vi "Time.vi"(8 "error in (no error)":errorcluster, 10 "Control In":T2={"I-O.lvclass"=refnum, "Gantry"=refnum, "Dispenser"="COM1"}, 11 "Sensor Dispense in":refnum<class "Sensor Dispense.lvclass">) -> (0 "error out":errorcluster, 1 "Timing Data":i32[](array[numeric]), 2 "Control Out":T2={"I-O.lvclass"=refnum, "Gantry"=refnum, "Dispenser"="COM1"}, 3 "Sensor Dispense out":refnum<class "Sensor Dispense.lvclass">)   [LabVIEW 2021, in "Sensor Dispense.lvclass"]
uses:
  Projects/Sensor Dispense.lvclass
  C:/Users/hep/Documents/UCSB-CMU-GantryCode/UCSB-Gantry-HEP-main (3)/UCSB-Gantry-HEP-main/Classes/Routine/Dispense/Dispense.lvclass
  Controller/Controllers.ctl
  Controller/I-O/I-O.lvclass
  C:/Program Files (x86)/Aerotech/A3200/LabVIEW/2010/Bin/Aerotech.A3200.dll
  Program Files (x86)/Aerotech/A3200/LabVIEW/2010/Bin/Aerotech.A3200.dll
  TypeOfHexaboard.ctl
  Projects/Sensor Dispense.lvclass/Sensor Dispense.ctl
  Controller/Motion/Motion.lvclass
  Controller/Motion/A3200/A3200.lvclass
  Controller/Controller.lvclass
  Routine.lvclass
panel:
  in  "Type of Hexaboard":T1
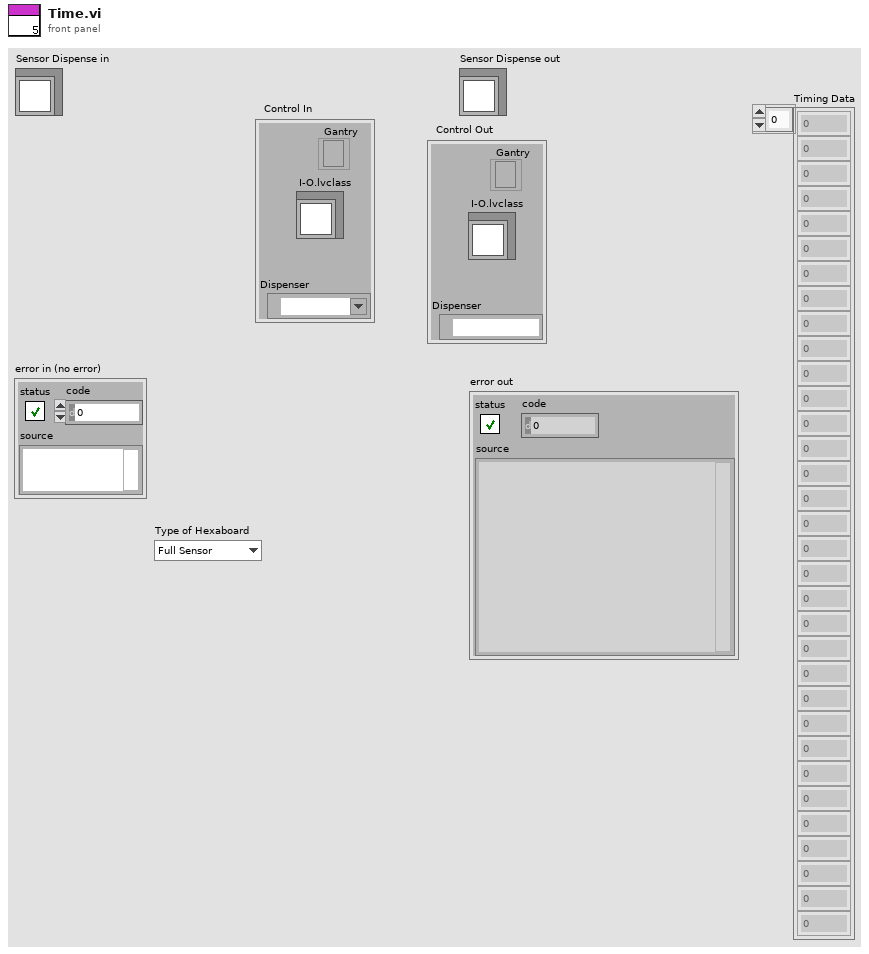
[diagram p1: front panel]
types:
  T1 = typedef "Routine.lvclass/TypeOfHexaboard.ctl" = enum16{"Full Sensor", "Full PCB", "Right Partial PCB", "Right Partial Sensor", "Al Dummy Right Partial Sensor"}
  T2 = typedef "Controller.lvclass/Controllers.ctl" = cluster{"I-O.lvclass":refnum<class "I-O.lvclass">, "Gantry":refnum<k24>, "Dispenser":refnum<visa-resource-name>}
  T3 = cluster{"Endpoints":dbl[][], "Center":dbl[], "CW/CCW":dbl, "Dispense Type":enum16{"N-gon", "Square", "Arc", "Dot", "Line", "Circle"}}[]
  T4 = cluster{"Endpoints":dbl[][], "Center":dbl[], "CW/CCW":dbl, "Dispense Type":enum16{"N-gon", "Square", "Arc", "Dot", "Line", "Circle"}}
  T5 = enum16{"N-gon", "Square", "Arc", "Dot", "Line", "Circle"}
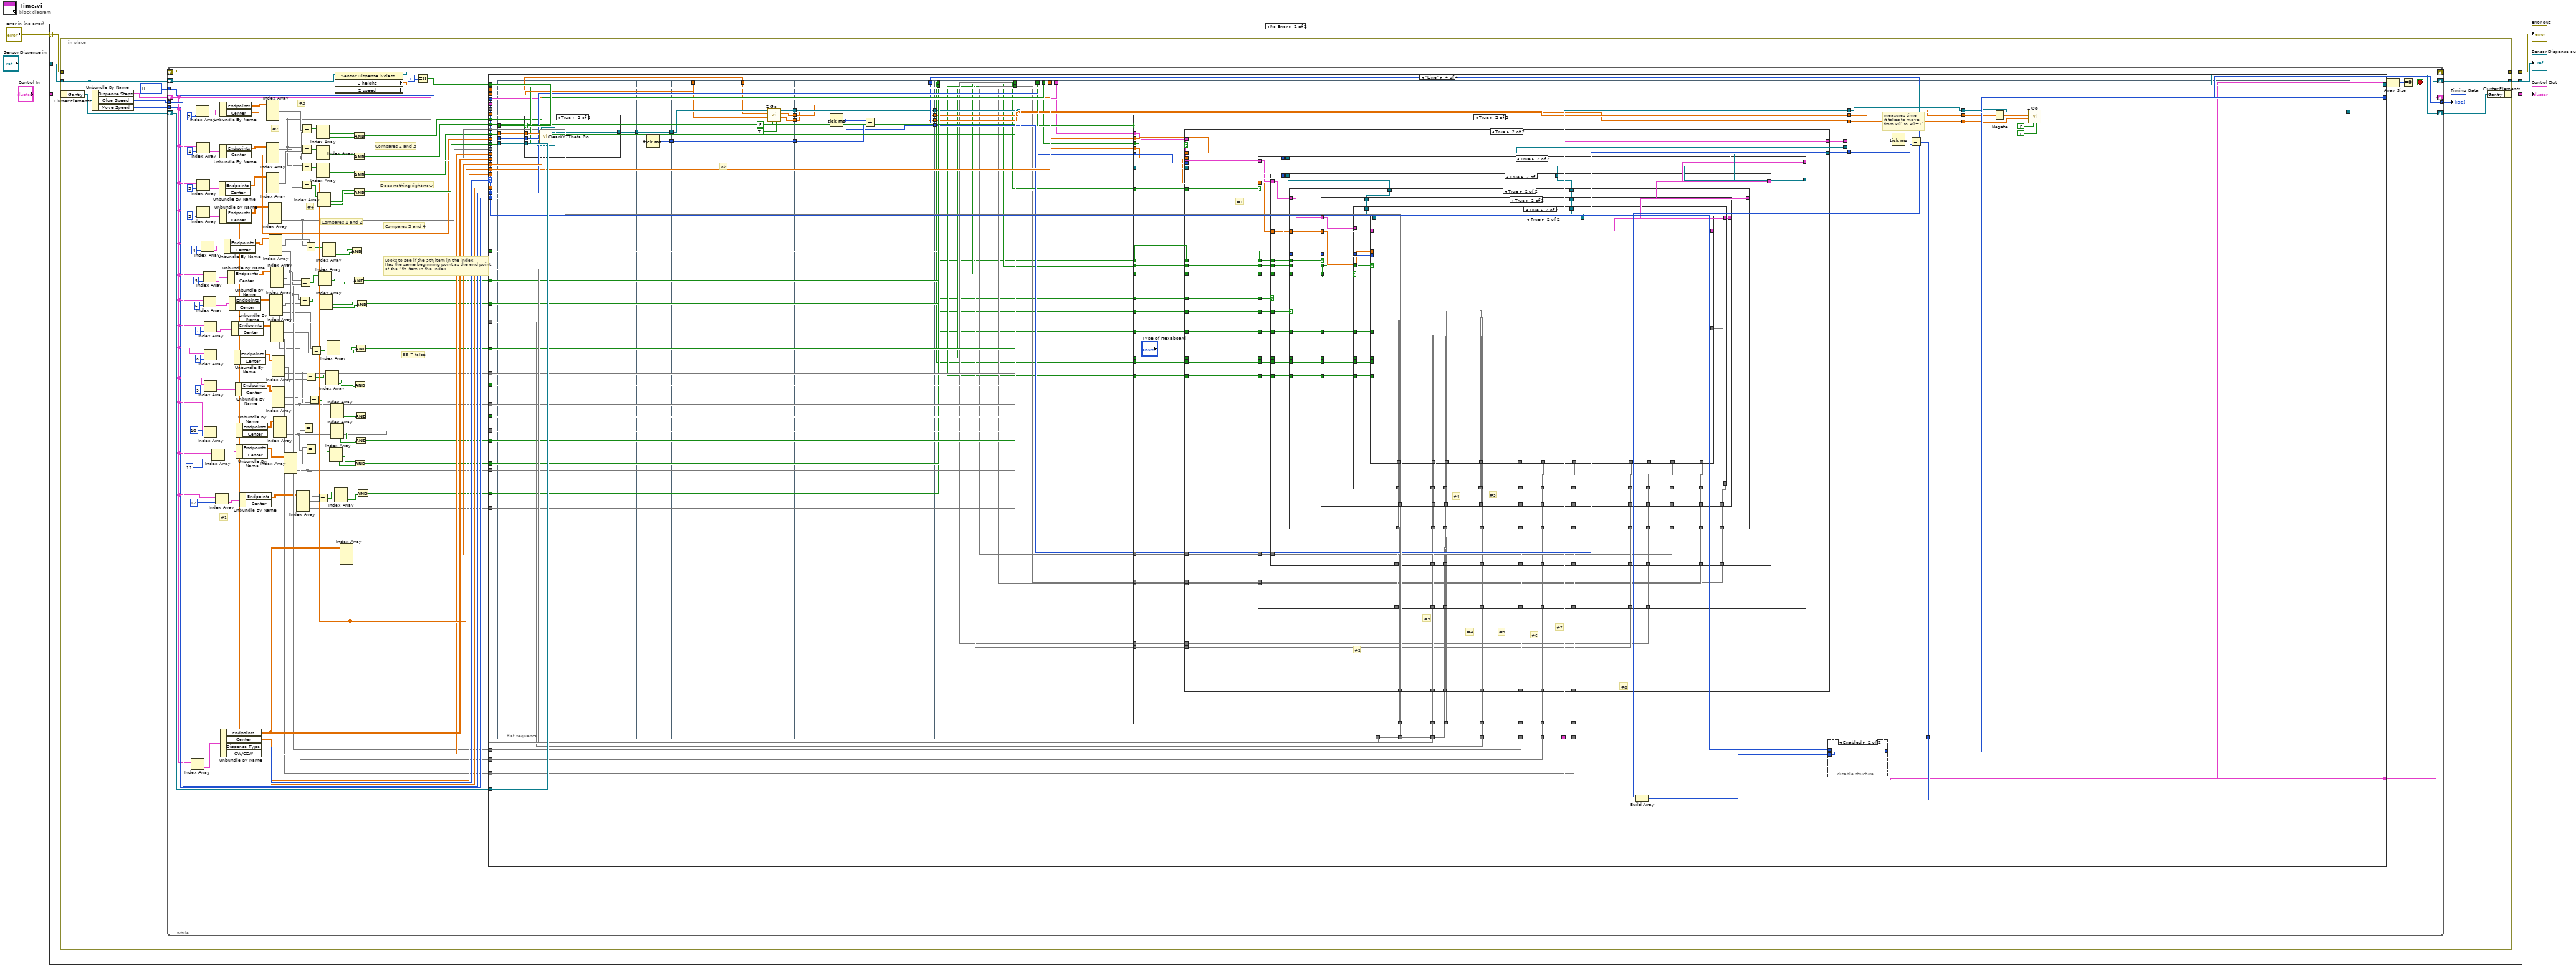
[diagram p0: block diagram]
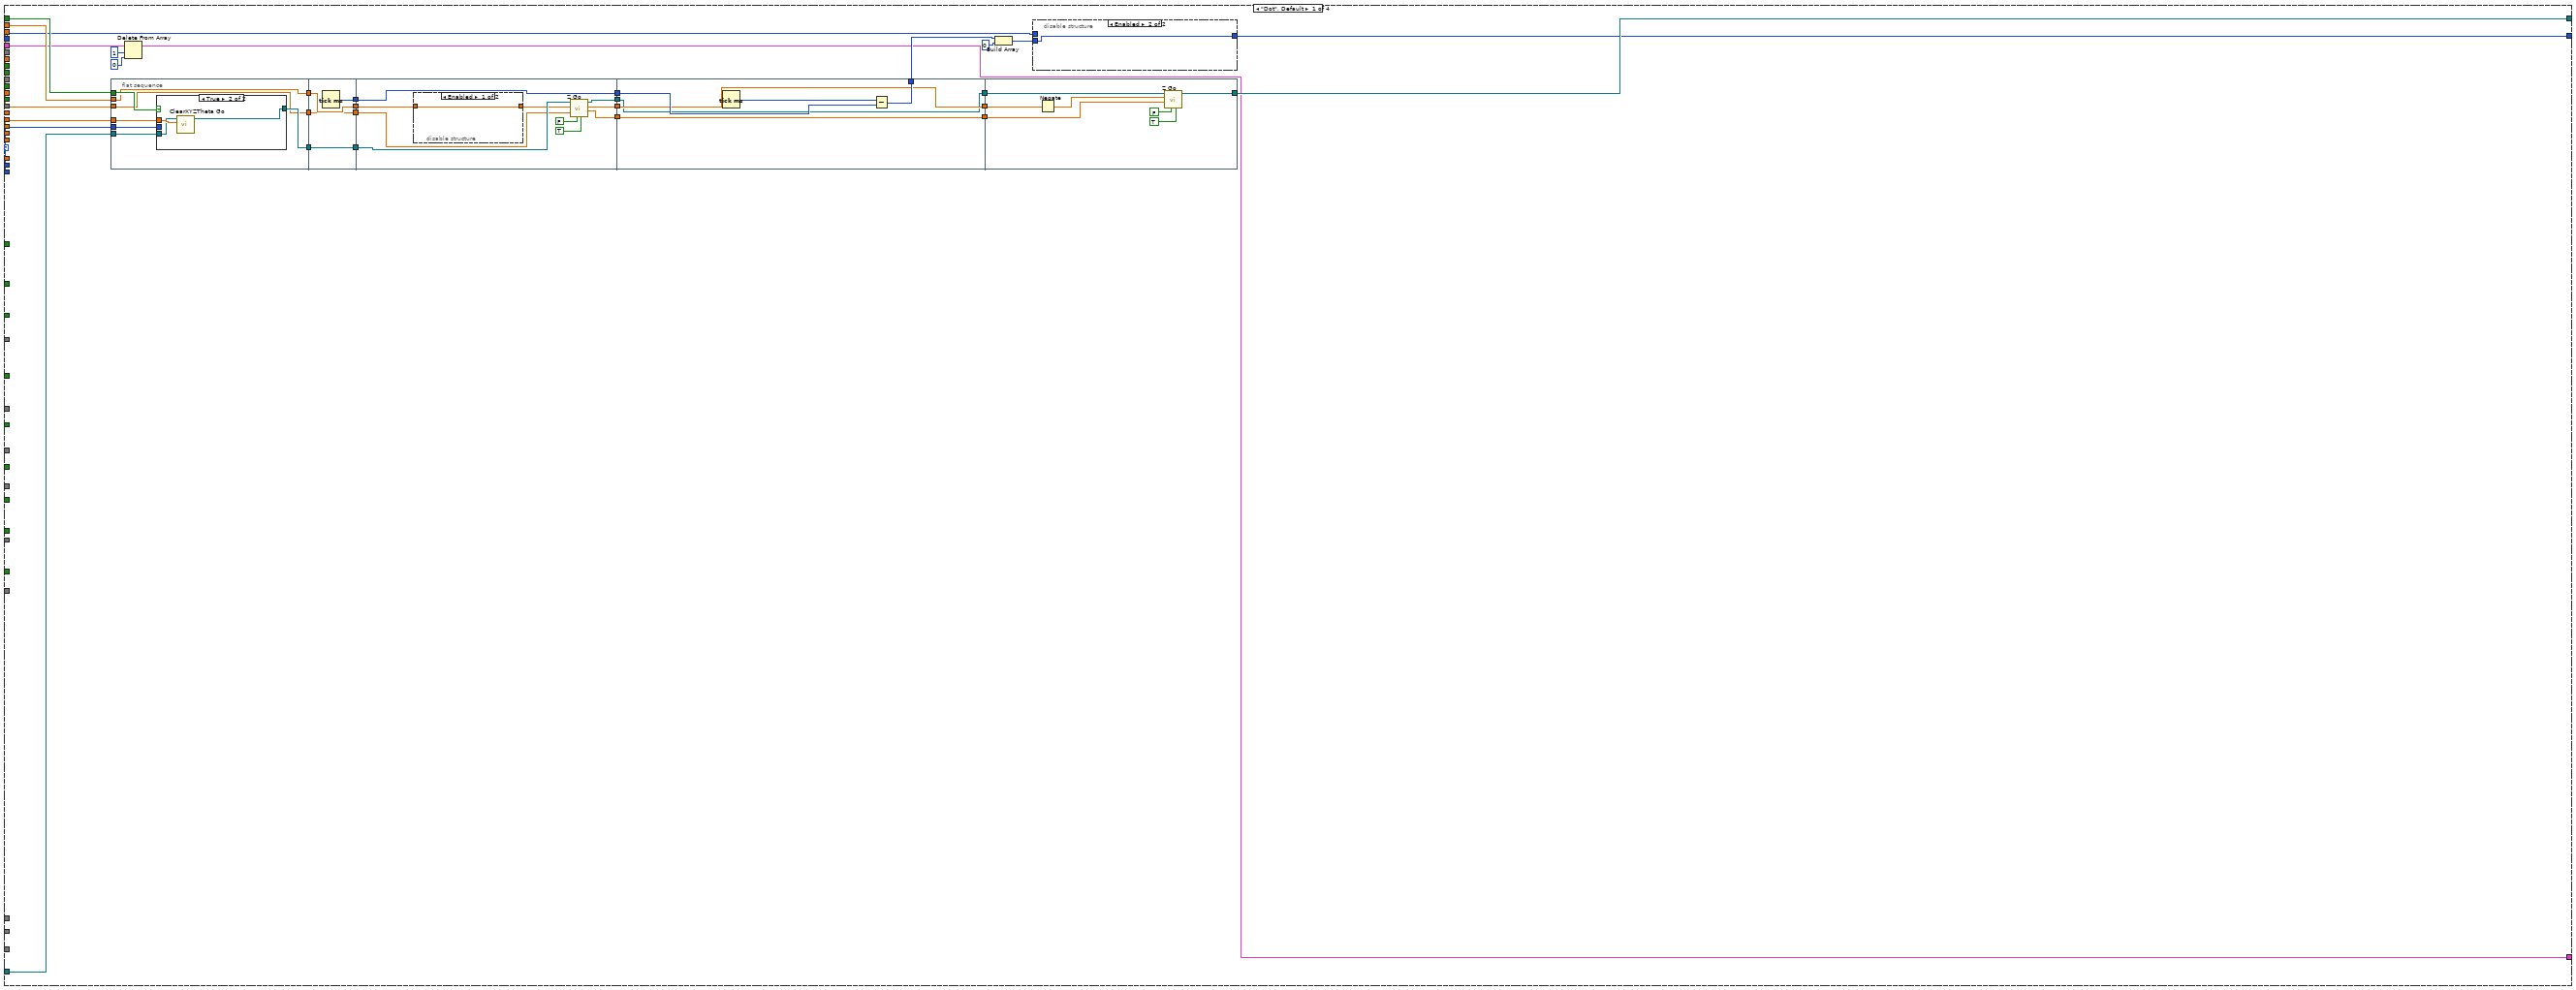
[diagram p2: hidden frame]
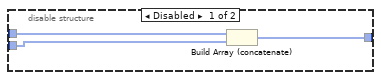
[diagram p3: hidden frame]
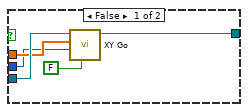
[diagram p4: hidden frame]
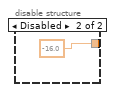
[diagram p5: hidden frame]
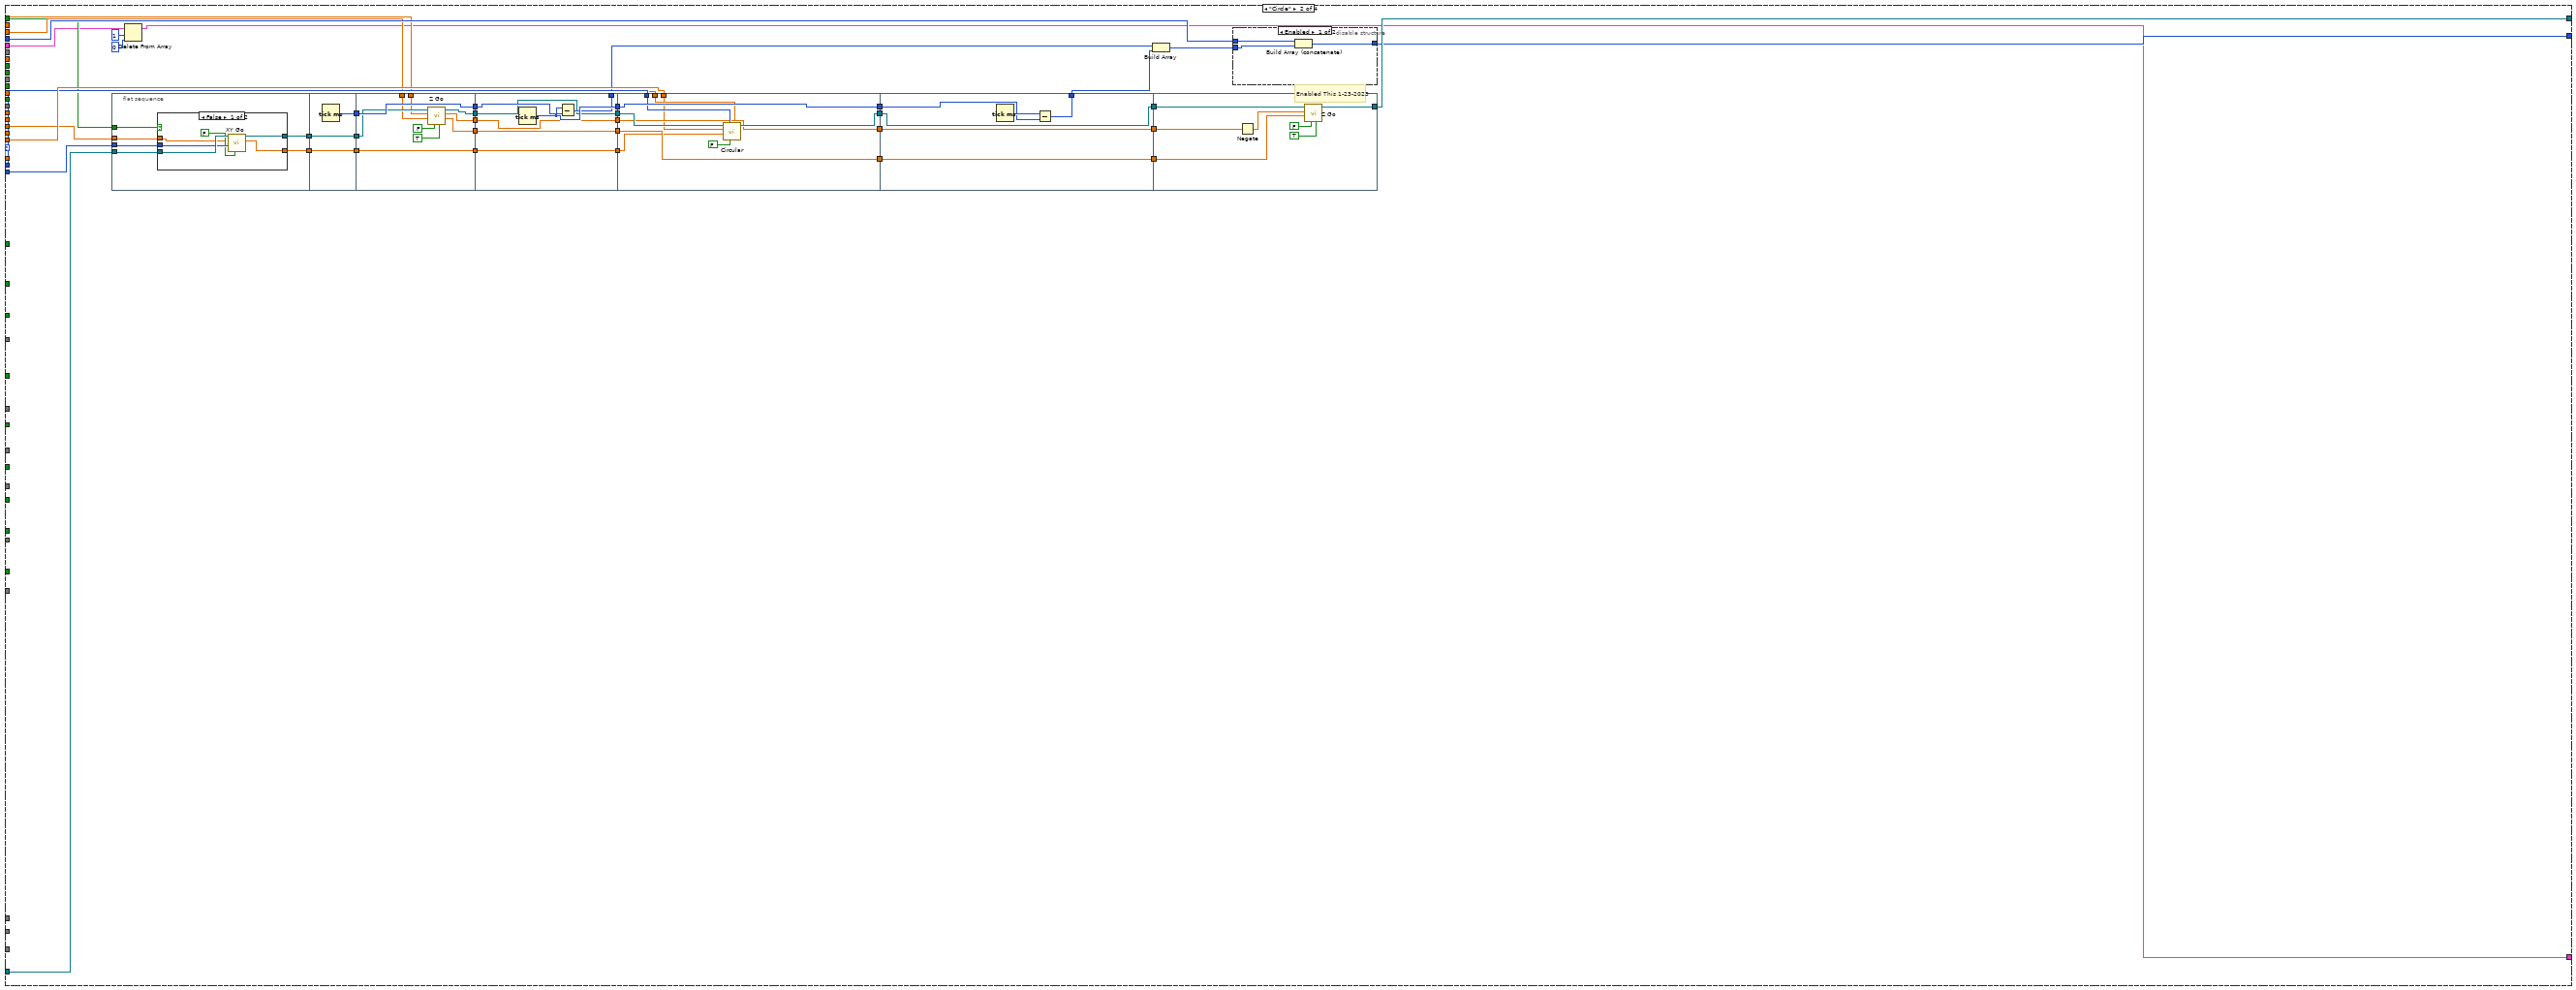
[diagram p6: hidden frame]
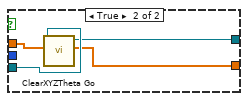
[diagram p8: hidden frame]
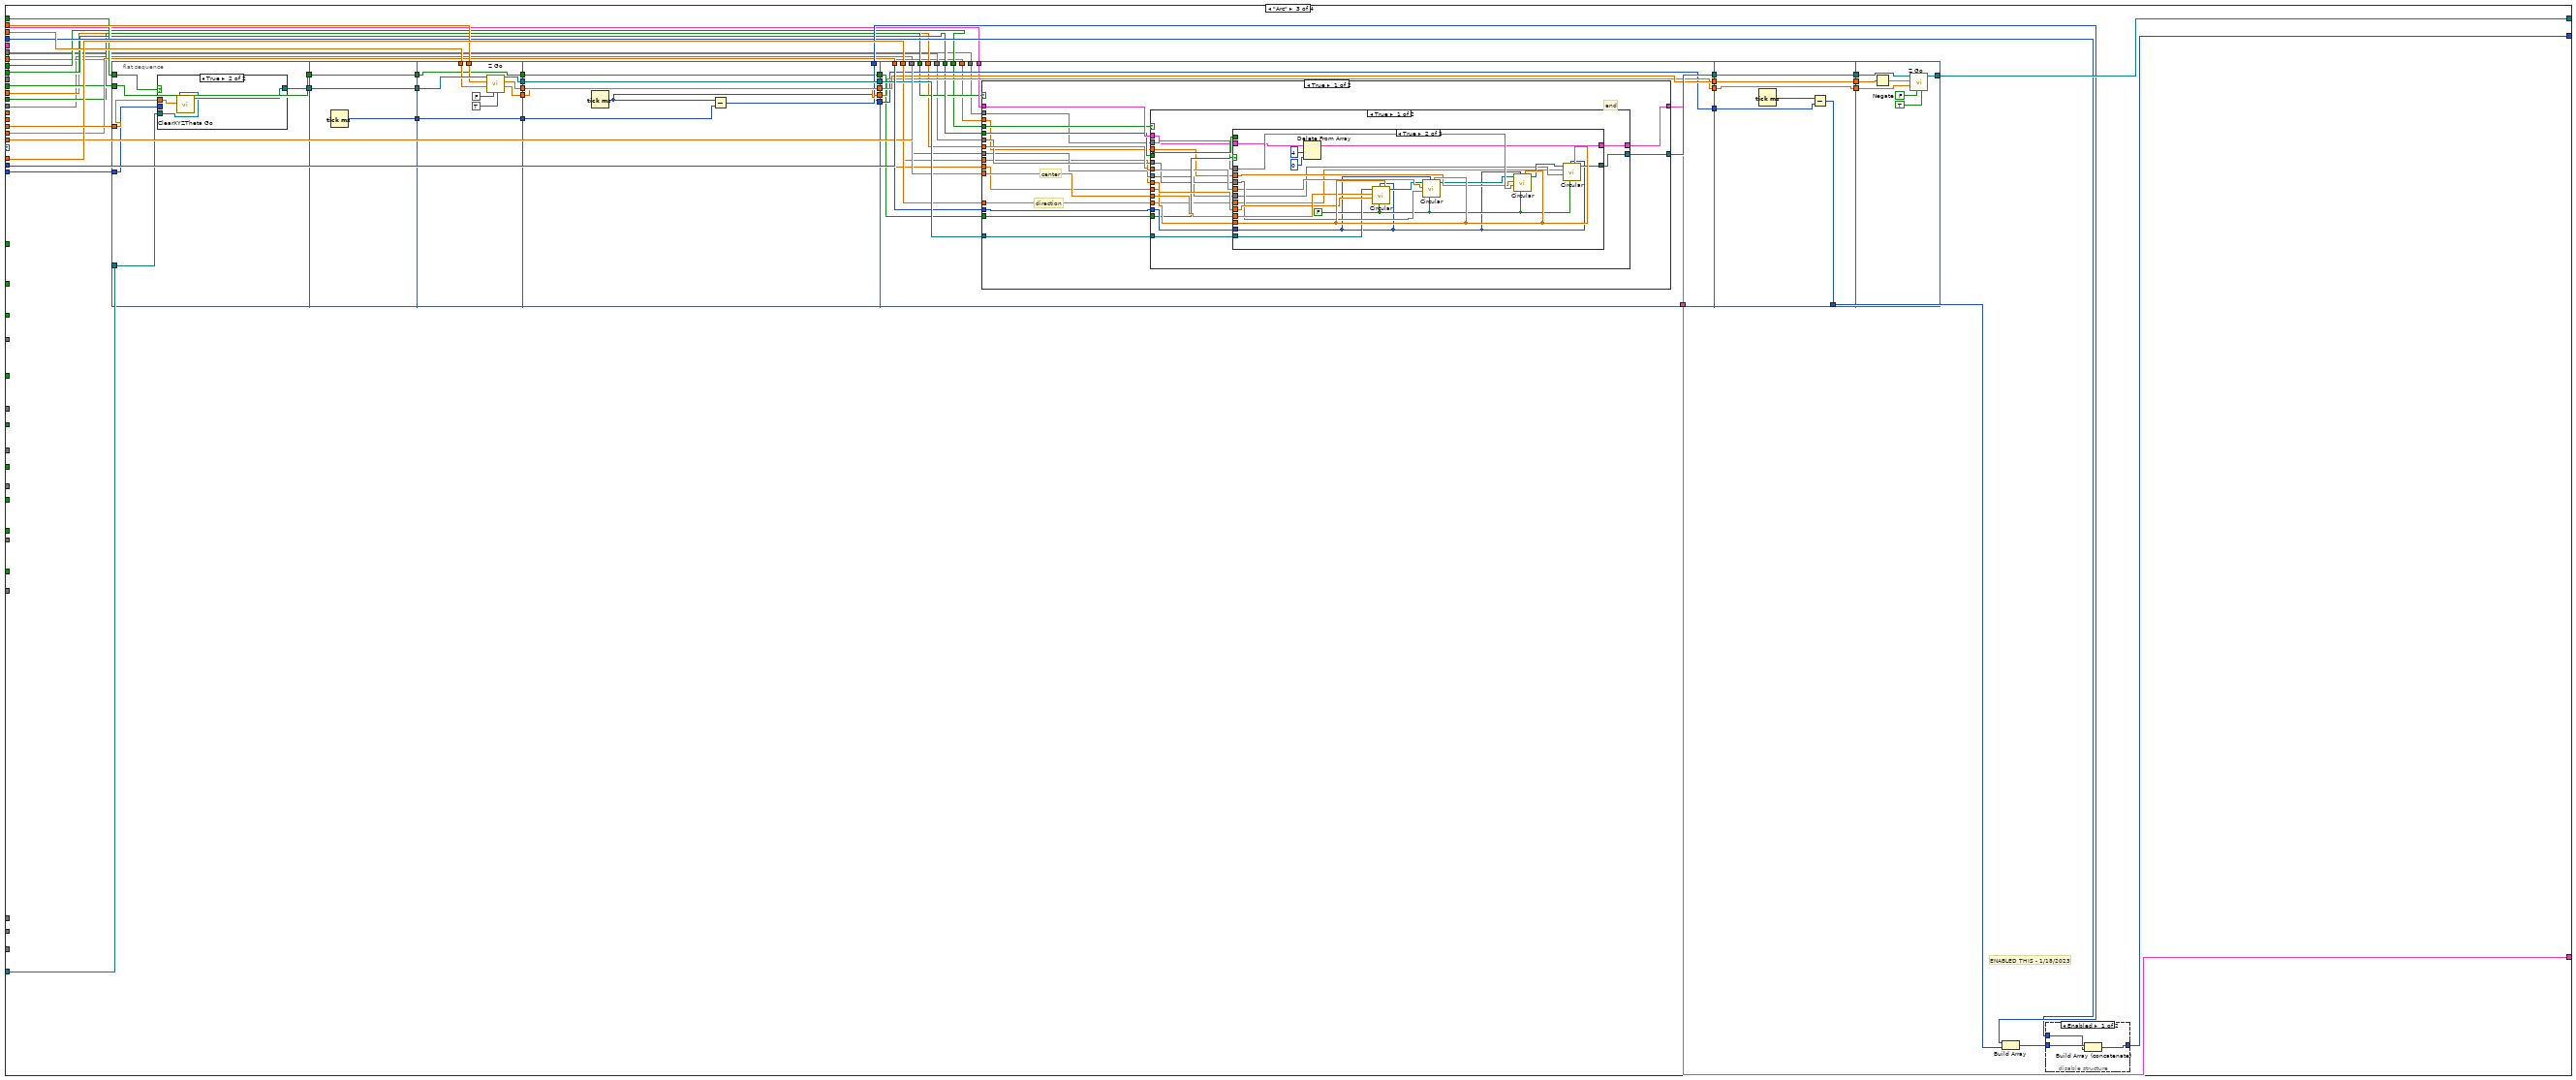
[diagram p9: hidden frame]
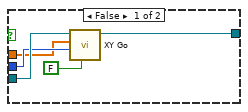
[diagram p11: hidden frame]
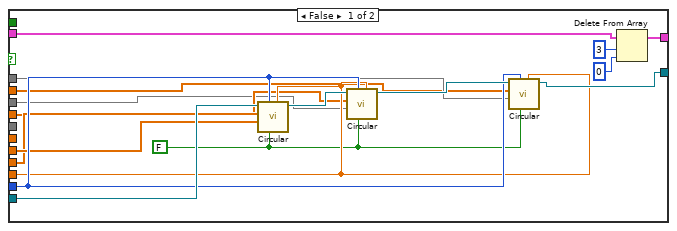
[diagram p12: hidden frame]
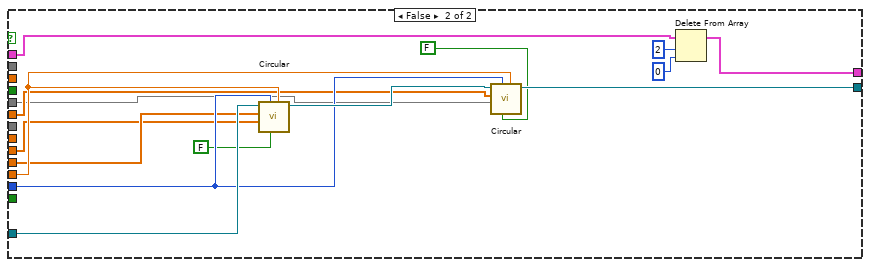
[diagram p13: hidden frame]
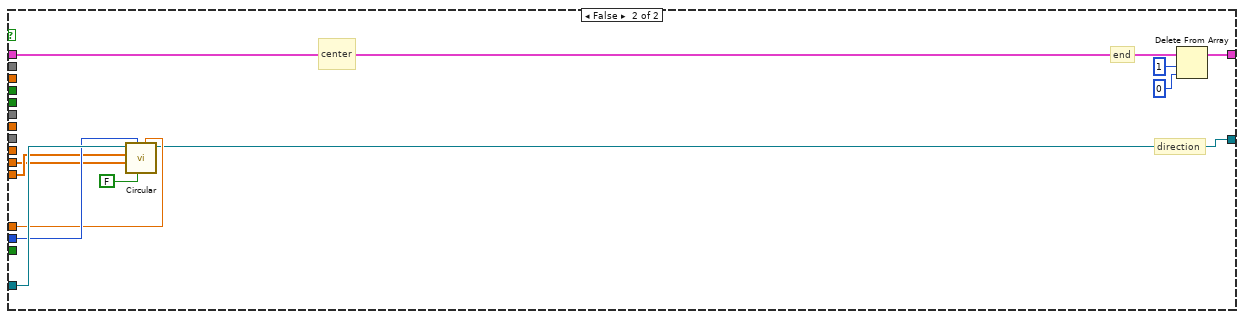
[diagram p14: hidden frame]
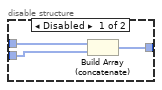
[diagram p15: hidden frame]
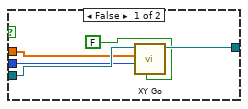
[diagram p16: hidden frame]
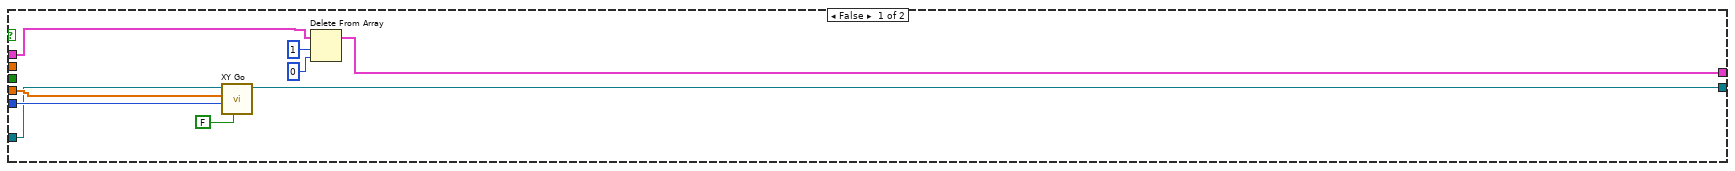
[diagram p17: hidden frame]
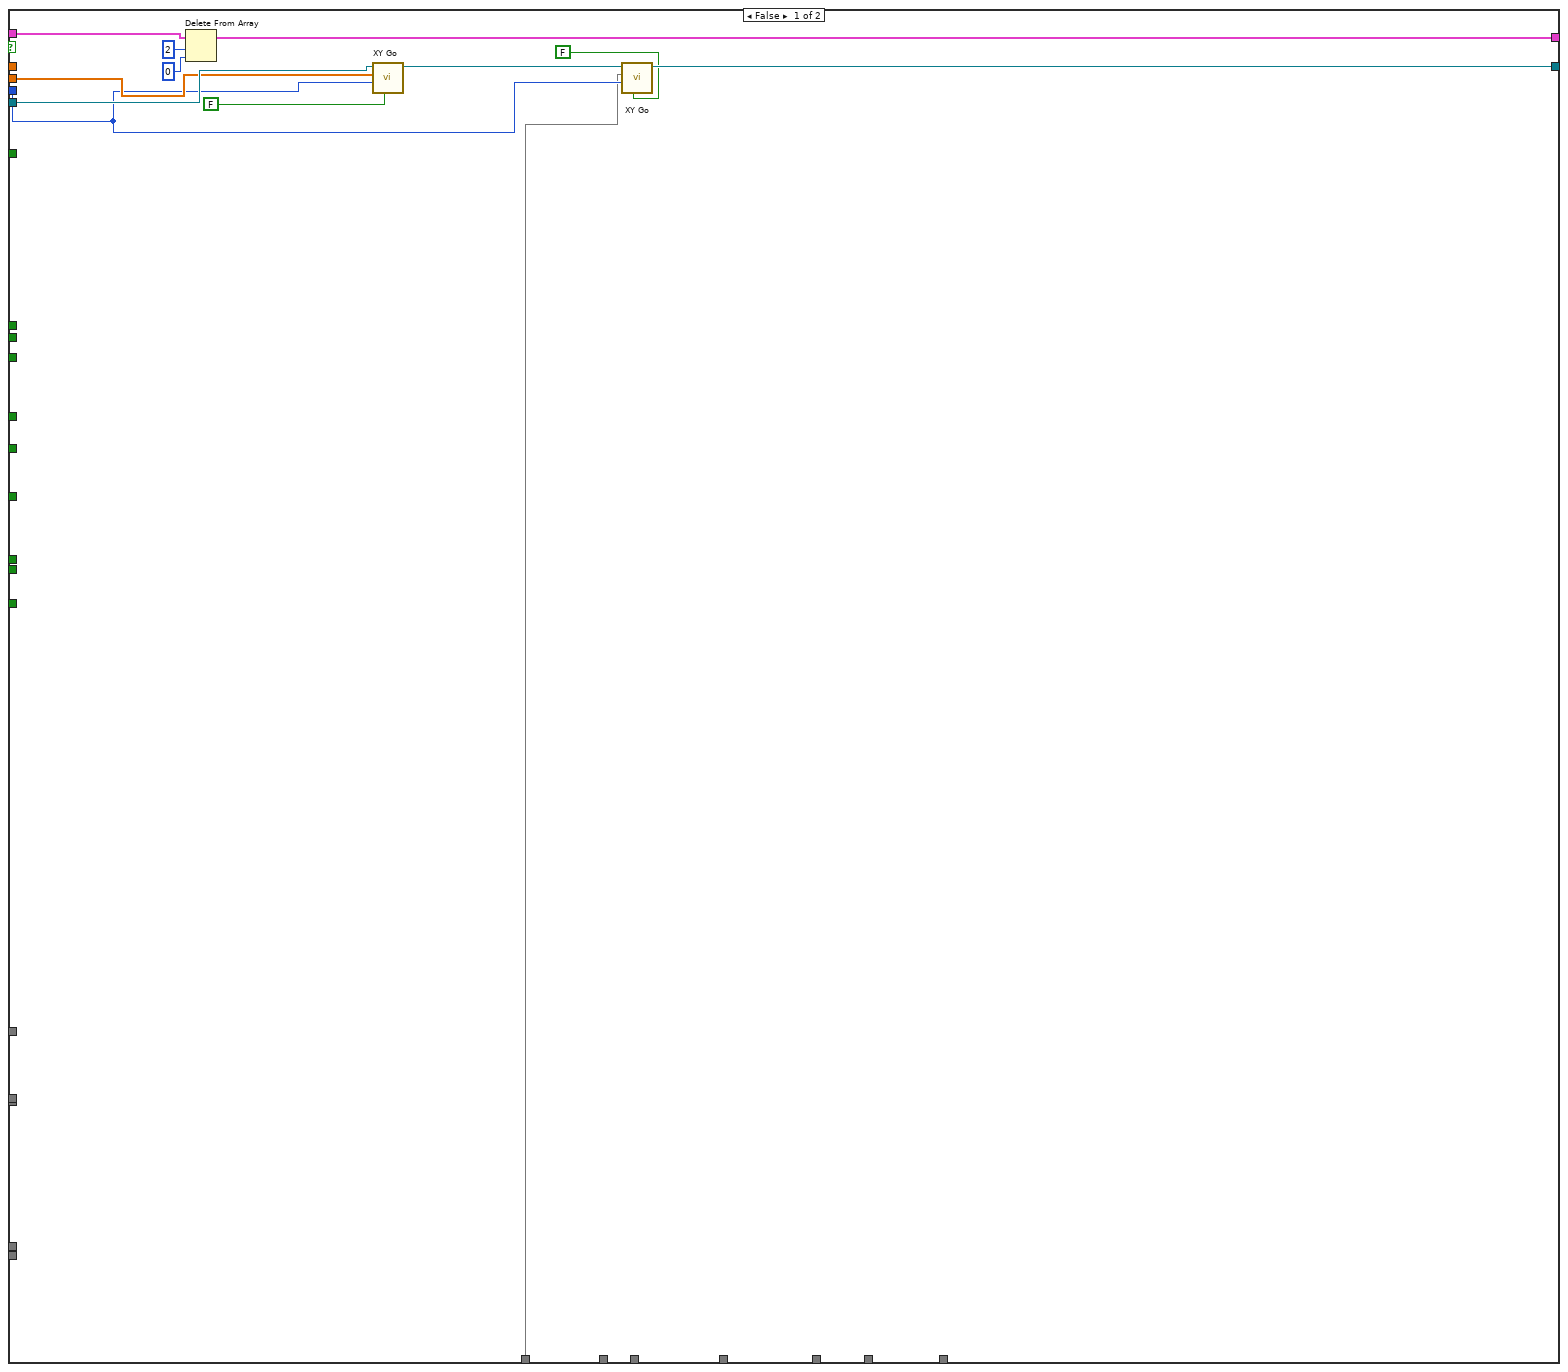
[diagram p18: hidden frame]
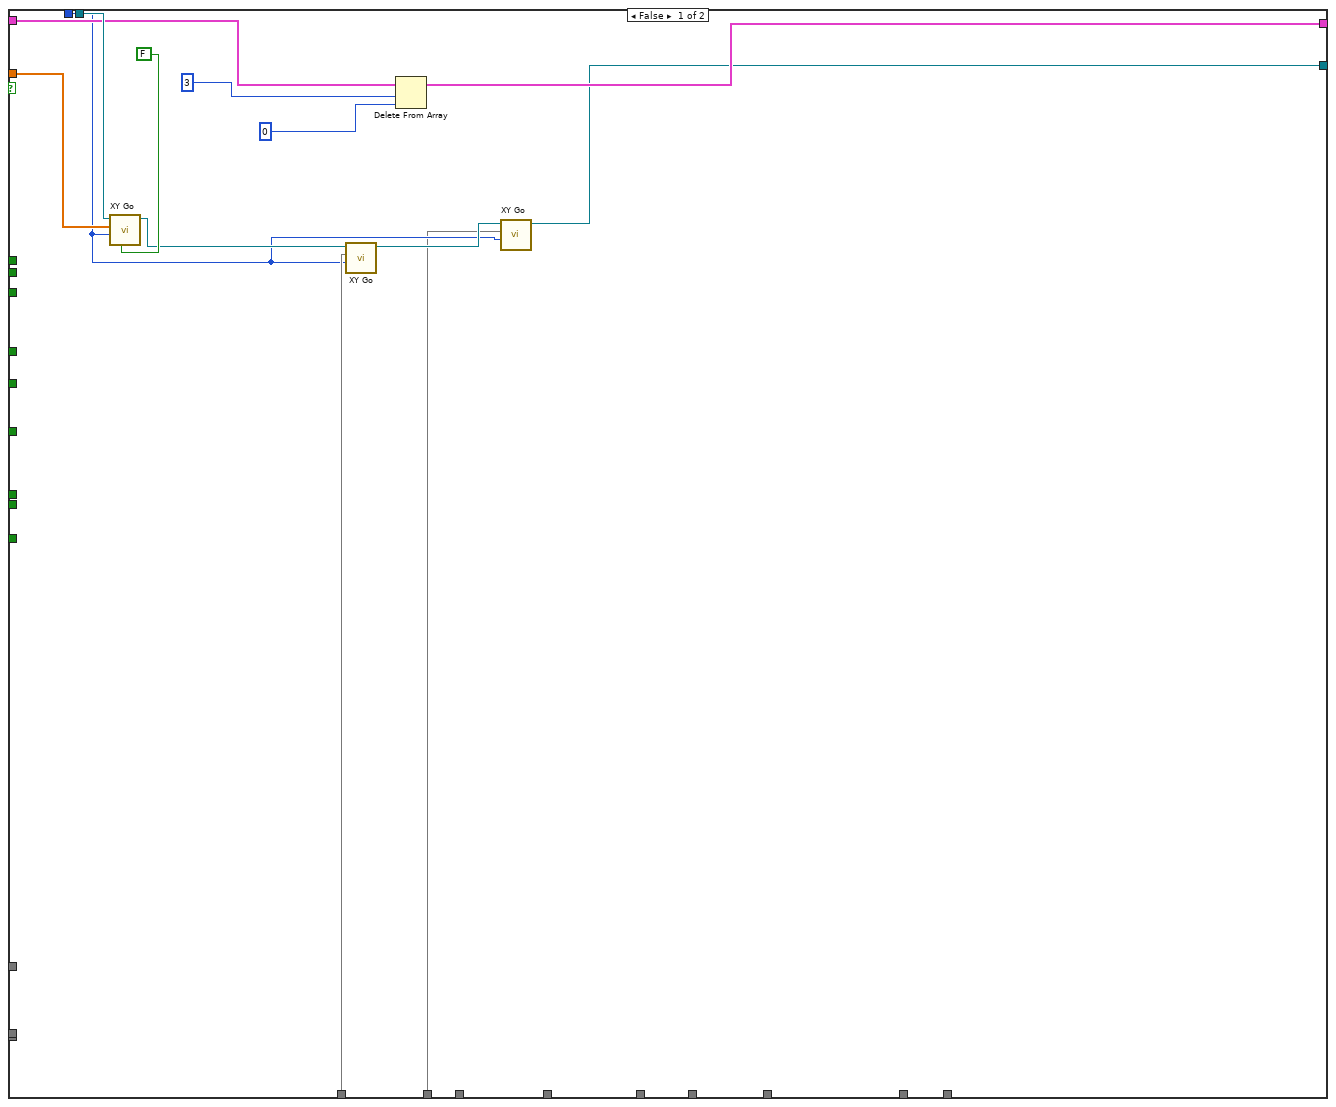
[diagram p19: hidden frame]
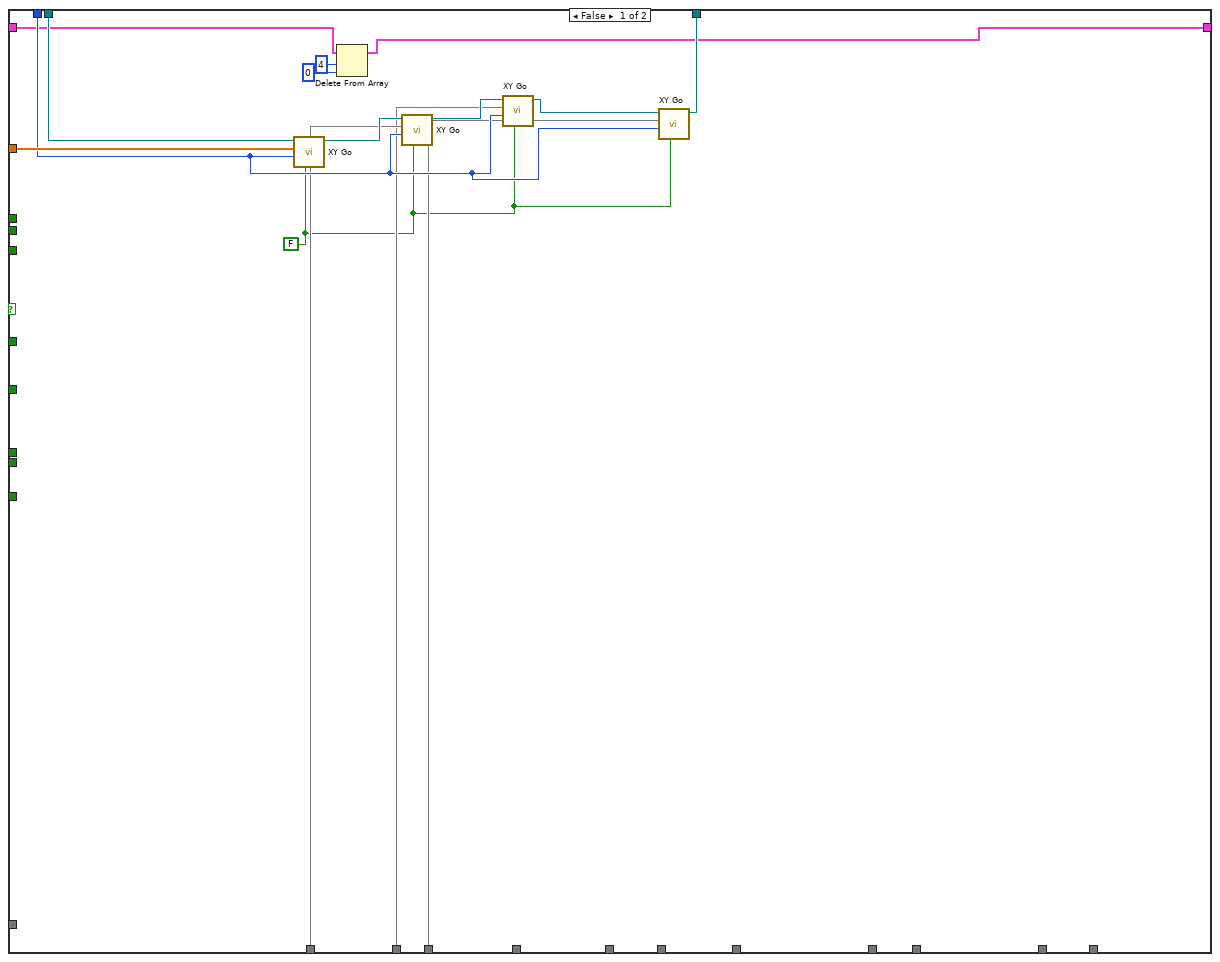
[diagram p20: hidden frame]
diagram:
  n1 = case shown="No Error" "error in (no error)" {
    selector: "error in (no error)" -> [w7 w1242]
    tunnel: "Sensor Dispense in" -> [w12 w1240]
    tunnel: [w11 w1240] -> w5
    tunnel: "Control In" -> [w10 w1241]
    tunnel: [w9 w1241] -> w3
    tunnel: [w8 w1242] -> w2
    frame No Error {
      n2 = in-place {
        in-place-border: w12 -> [w21]
        in-place-border: [w20] -> w11
        in-place-border: [w16] -> w8
        in-place-border: w7 -> [w15]
        n3 = in-place-cluster #1(w10) -> ("Gantry"=w22:refnum<k24>)
        n4 = Unbundle By Name "Unbundle By Name"(w21) -> ("Dispense Steps"=w17:T3, "Glue Speed"=w13:i32, "Move Speed"=w14:i32)
        n5 = while {
          tunnel: w14 -> [w166]
          shift-right: [w155] -> w19
          shift-left: w22 -> [w164]
          tunnel: w13 -> [w152]
          shift-right: [w162] -> w20
          shift-left: w21 -> [w163]
          shift-right: [w113] -> w16
          shift-left: w15 -> [w113]
          tunnel: i32[] [] -> [w165]
          tunnel: [w157] -> w18 mode=concatenating
          shift-right: [w115] -> _
          shift-left: w17 -> [w40]
          i -> [w161]
          stop <- w112 stop-if-true
          # "85 = false"
          # "Looks to see if the 5th item in the index\nHas the same beginning point as the end point\nof the 4th item in the index"
          # "Does nothing right now"
          # "Compares 2 and 3"
          # "Compares 3 and 4"
          # "Compares 1 and 2"
          # "#3"
          # "#2"
          # "#1"
          # "#4"
          n6 = Index Array(array=w40) -> (element=w148:T4)  [unwired: 1 in]
          n7 = Index Array "Index Array"(array=w40, index=2) -> (element=w146:T4)
          n8 = Index Array(array=w40, index=1) -> (element=w145:T4)
          n9 = Index Array(array=w40, index=3) -> (element=w147:T4)
          n10 = Index Array(array=w40, index=3) -> (element=w150:T4)
          n11 = Index Array "Index Array"(array=w40, index=4) -> (element=w105:T4)
          n12 = Index Array "Index Array"(array=w40, index=5) -> (element=w93:T4)
          n13 = Index Array "Index Array"(array=w40, index=6) -> (element=w94:T4)
          n14 = Index Array "Index Array"(array=w40, index=7) -> (element=w95:T4)
          n15 = Index Array "Index Array"(array=w40, index=8) -> (element=w70:T4)
          n16 = Index Array "Index Array"(array=w40, index=9) -> (element=w69:T4)
          n17 = Index Array "Index Array"(array=w40, index=10) -> (element=w68:T4)
          n18 = Index Array "Index Array"(array=w40, index=11) -> (element=w67:T4)
          n19 = Index Array "Index Array"(array=w40, index=12) -> (element=w66:T4)
          n20 = Unbundle By Name(w147) -> ("Endpoints"=w139:dbl[][])  [unwired: 1 out]
          n21 = Unbundle By Name(w146) -> ("Endpoints"=w140:dbl[][], "Center"=w117:dbl[])
          n22 = Unbundle By Name(w145) -> ("Endpoints"=w138:dbl[][], "Center"=w109:dbl[])
          n23 = Unbundle By Name(w150) -> ("Endpoints"=w141:dbl[][], "Center"=w116:dbl[])
          n24 = Unbundle By Name(w148) -> ("Endpoints"=w154:dbl[][], "Center"=w153:dbl[], "Dispense Type"=w156:T5, "CW/CCW"=w151:dbl)
          n25 = Unbundle By Name(w105) -> ("Endpoints"=w101:dbl[][])  [unwired: 1 out]
          n26 = Unbundle By Name(w93) -> ("Endpoints"=w92:dbl[][])  [unwired: 1 out]
          n27 = Unbundle By Name(w94) -> ("Endpoints"=w91:dbl[][])  [unwired: 1 out]
          n28 = Unbundle By Name(w95) -> ("Endpoints"=w90:dbl[][])  [unwired: 1 out]
          n29 = Unbundle By Name(w70) -> ("Endpoints"=w65:dbl[][])  [unwired: 1 out]
          n30 = Unbundle By Name(w69) -> ("Endpoints"=w60:dbl[][])  [unwired: 1 out]
          n31 = Unbundle By Name(w68) -> ("Endpoints"=w54:dbl[][])  [unwired: 1 out]
          n32 = Unbundle By Name(w67) -> ("Endpoints"=w48:dbl[][])  [unwired: 1 out]
          n33 = Unbundle By Name(w66) -> ("Endpoints"=w42:dbl[][])  [unwired: 1 out]
          n34 = Index Array(array=w140) -> (element #1=w130:dbl[], element #2=w118:dbl[])  [unwired: 4 in]
          n35 = Index Array(array=w138) -> (element #1=w121:dbl[], element #2=w111:dbl[])  [unwired: 4 in]
          n36 = Index Array(array=w139) -> (element #1=w134:dbl[])  [unwired: 4 in, 1 out]
          n37 = Index Array(array=w141) -> (element #1=w123:dbl[], element #2=w99:dbl[])  [unwired: 4 in]
          n38 = Index Array(array=w101) -> (element #1=w100:dbl[], element #2=w89:dbl[])  [unwired: 4 in]
          n39 = Index Array(array=w91) -> (element #1=w83:dbl[], element #2=w38:dbl[])  [unwired: 4 in]
          n40 = Index Array(array=w92) -> (element #1=w88:dbl[], element #2=w84:dbl[])  [unwired: 4 in]
          n41 = Index Array(array=w90) -> (element #1=w79:dbl[], element #2=w39:dbl[])  [unwired: 4 in]
          n42 = Index Array(array=w65) -> (element #1=w64:dbl[], element #2=w58:dbl[])  [unwired: 4 in]
          n43 = Index Array(array=w60) -> (element #1=w59:dbl[], element #2=w53:dbl[])  [unwired: 4 in]
          n44 = Index Array(array=w54) -> (element #1=w52:dbl[], element #2=w46:dbl[])  [unwired: 4 in]
          n45 = Index Array(array=w48) -> (element #1=w47:dbl[], element #2=w32:dbl[])  [unwired: 4 in]
          n46 = Index Array(array=w42) -> (element #1=w33:dbl[], element #2=w41:dbl[])  [unwired: 4 in]
          n47 = Equal?(x=w84, y=w83) -> (x = y?=w82:bool[])
          n48 = Equal?(x=w89, y=w88) -> (x = y?=w87:bool[])
          n49 = Equal?(x=w111, y=w130) -> (x = y?=w129:bool[])
          n50 = Equal?(x=w118, y=w134) -> (x = y?=w133:bool[])
          n51 = Equal?(x=w118, y=w123) -> (x = y?=w137:bool[])
          n52 = Equal?(x=w52, y=w53) -> (x = y?=w51:bool[])
          n53 = Equal?(x=w99, y=w100) -> (x = y?=w102:bool[])
          n54 = Equal?(x=w39, y=w64) -> (x = y?=w63:bool[])
          n55 = Equal?(x=w47, y=w46) -> (x = y?=w45:bool[])
          n56 = Equal?(x=w59, y=w58) -> (x = y?=w57:bool[])
          n57 = Equal?(x=w38, y=w79) -> (x = y?=w78:bool[])
          n58 = Index Array(array=w129) -> (element #1=w128:bool, element #2=w127:bool)  [unwired: 2 in]
          n59 = Index Array(array=w133) -> (element #1=w132:bool, element #2=w131:bool)  [unwired: 2 in]
          n60 = Index Array(array=w137) -> (element #1=w136:bool, element #2=w135:bool)  [unwired: 2 in]
          n61 = Equal?(x=w32, y=w33) -> (x = y?=w31:bool[])
          n62 = Index Array(array=w87) -> (element #1=w86:bool, element #2=w85:bool)  [unwired: 2 in]
          n63 = Index Array(array=w82) -> (element #1=w81:bool, element #2=w80:bool)  [unwired: 2 in]
          n64 = Index Array(array=w102) -> (element #1=w104:bool, element #2=w103:bool)  [unwired: 2 in]
          n65 = Index Array(array=w63) -> (element #1=w62:bool, element #2=w61:bool)  [unwired: 2 in]
          n66 = Index Array(array=w78) -> (element #1=w77:bool, element #2=w76:bool)  [unwired: 2 in]
          n67 = Index Array(array=w45) -> (element #1=w44:bool, element #2=w43:bool)  [unwired: 2 in]
          n68 = Index Array(array=w57) -> (element #1=w56:bool, element #2=w55:bool)  [unwired: 2 in]
          n69 = Index Array(array=w51) -> (element #1=w50:bool, element #2=w49:bool)  [unwired: 2 in]
          n70 = Index Array(array=w31) -> (element #1=w30:bool, element #2=w29:bool)  [unwired: 2 in]
          n71 = property class="Sensor Dispense.lvclass"(reference=w163) -> (reference out=w162:refnum<class "Sensor Dispense.lvclass">, "Z height"=w159:dbl, "Z speed"=w158:dbl)  [unwired: 1 in, 1 out]
          n72 = Index Array(array=w154) -> (element #1=w110:dbl[], element #2=w122:dbl[])  [unwired: 4 in]
          n73 = Equal?(x=w122, y=w121) -> (x = y?=w126:bool[])
          n74 = Index Array(array=w126) -> (element #1=w125:bool, element #2=w124:bool)  [unwired: 2 in]
          n75 = And(x=w104, y=w103) -> (x .and. y?=w25:bool)
          n76 = And(x=w86, y=w85) -> (x .and. y?=w24:bool)
          n77 = And(x=w128, y=w127) -> (x .and. y?=w120:bool)
          n78 = And(x=w132, y=w131) -> (x .and. y?=w107:bool)
          n79 = And(x=w136, y=w135) -> (x .and. y?=w108:bool)
          n80 = And(x=w125, y=w124) -> (x .and. y?=w119:bool)
          n81 = And(x=w62, y=w61) -> (x .and. y?=w36:bool)
          n82 = And(x=w44, y=w43) -> (x .and. y?=w28:bool)
          n83 = And(x=w77, y=w76) -> (x .and. y?=w37:bool)
          n84 = And(x=w56, y=w55) -> (x .and. y?=w35:bool)
          n85 = And(x=w50, y=w49) -> (x .and. y?=w34:bool)
          n86 = And(x=w81, y=w80) -> (x .and. y?=w26:bool)
          n87 = And(x=w30, y=w29) -> (x .and. y?=w27:bool)
          n88 = Equal To 0?(x=w161) -> (x = 0?=w160:bool)
          n89 = case shown="\"Line\"" w156 {
            tunnel: w153 -> [_ w273 w373 _]
            tunnel: w164 -> [w192 w274 w398 w626]
            tunnel: w166 -> [w176 w262 w396 w624]
            tunnel: [w177 w281 w385 w600] -> w155
            tunnel: w152 -> [_ w272 w395 w614]
            tunnel: w151 -> [_ w271 w394 _]
            tunnel: w165 -> [w173 w268 w377 w598]
            tunnel: [w171 w266 w376 w596] -> w157
            tunnel: w110 -> [w193 w261 w397 w625]
            tunnel: w158 -> [w186 w264 w392 w619]
            tunnel: w159 -> [w189 w265 w393 w620]
            tunnel: w160 -> [w194 w263 w375 w623]
            tunnel: w154 -> [_ _ _ _]
            tunnel: w122 -> [_ _ w374 w595]
            tunnel: w40 -> [w170 w248 w364 w591]
            tunnel: [w169 w247 w363 w590] -> w115
            tunnel: w108 -> [_ _ w358 w587]
            tunnel: w107 -> [_ _ w357 w586]
            tunnel: w120 -> [_ _ w356 w593]
            tunnel: w119 -> [_ _ w355 w594]
            tunnel: w109 -> [_ _ w354 _]
            tunnel: w111 -> [_ _ w353 w589]
            tunnel: w118 -> [_ _ w352 w588]
            tunnel: w117 -> [_ _ w351 w592]
            tunnel: w99 -> [_ _ w350 w585]
            tunnel: w116 -> [_ _ w349 _]
            tunnel: w89 -> [_ _ _ w584]
            tunnel: w84 -> [_ _ _ w583]
            tunnel: w38 -> [_ _ _ w582]
            tunnel: w39 -> [_ _ _ w581]
            tunnel: w58 -> [_ _ _ w580]
            tunnel: w53 -> [_ _ _ w579]
            tunnel: w46 -> [_ _ _ w578]
            tunnel: w32 -> [_ _ _ w577]
            tunnel: w41 -> [_ _ _ w576]
            tunnel: w37 -> [_ _ _ w575]
            tunnel: w36 -> [_ _ _ w574]
            tunnel: w35 -> [_ _ _ w573]
            tunnel: w34 -> [_ _ _ w572]
            tunnel: w28 -> [_ _ _ w571]
            tunnel: w27 -> [_ _ _ w570]
            tunnel: w26 -> [_ _ _ w569]
            tunnel: w25 -> [_ _ _ w568]
            tunnel: w24 -> [_ _ _ w567]
            frame "Dot", Default {
              n90 = flat-sequence {
                tunnel: w194 -> [w207]
                tunnel: w193 -> [w206]
                tunnel: w192 -> [w205]
                tunnel: [w204] -> w190
                tunnel: w189 -> [w203]
                tunnel: [w203] -> w187
                tunnel: w186 -> [w202]
                tunnel: [w202] -> w184
                tunnel: w176 -> [w201]
                tunnel: [w219] -> w196
                tunnel: [w218] -> w191
                tunnel: w190 -> [w218]
                tunnel: [w217] -> w188
                tunnel: w187 -> [w217]
                tunnel: [w216] -> w185
                tunnel: w184 -> [w216]
                tunnel: [w229] -> w195
                tunnel: w196 -> [w229]
                tunnel: w191 -> [w228]
                tunnel: w188 -> [w221]
                tunnel: w185 -> [w227]
                tunnel: [w226] -> w182
                tunnel: [w225] -> w180
                tunnel: [w224] -> w178
                tunnel: w195 -> [w237]
                tunnel: [w235] -> w175
                tunnel: [w234] -> w183
                tunnel: w182 -> [w234]
                tunnel: [w233] -> w181
                tunnel: w180 -> [w233]
                tunnel: [w232] -> w179
                tunnel: w178 -> [w232]
                tunnel: w183 -> [w244]
                tunnel: w181 -> [w242]
                tunnel: w179 -> [w241]
                tunnel: [w240] -> w177
                frame #0 {
                  n91 = case shown="True" w207 {
                    tunnel: w206 -> [w210 w215]
                    tunnel: w205 -> [w212 w214]
                    tunnel: [w211 w213] -> w204
                    tunnel: w201 -> [w209 _]
                    frame False {
                      n92 = call "XY Go.vi"("return immediately"=FALSE, "Speed"=w209, "XY In"=w210, "Gantry In"=w212) -> ("Gantry Out"=w211:refnum<k24>)  [unwired: 5 in, 2 out]
                    }
                    frame True {
                      n93 = call "ClearXYZTheta Go.vi"("XYZTheta In"=w215, "Gantry In"=w214) -> ("Gantry Out"=w213:refnum<k24>)  [unwired: 7 in, 2 out]
                    }
                  }
                }
                frame #1 {
                  n94 = Tick Count (ms)() -> (millisecond timer value=w219:u32)
                }
                frame #2 {
                  n95 = disable-structure shown="Enabled" {
                    disable-tunnel: w221 -> [w230 _]
                    disable-tunnel: [w230 -16.0 ("Z height")] -> w220
                    frame Enabled {
                    }
                    frame Disabled {
                    }
                  }
                  n96 = call "Z Go.vi"("Increment"=TRUE, "Return Immediately"=FALSE, "Speed In"=w227, "Position In"=w220, "Gantry In"=w228) -> ("Speed Out"=w225:dbl, "Position Out"=w226:dbl, "Gantry Out"=w224:refnum<k24>)  [unwired: 3 in, 1 out]
                }
                frame #3 {
                  n97 = Tick Count (ms)() -> (millisecond timer value=w236:u32)
                  n98 = Subtract(x=w236, y=w237) -> (x-y=w235:u32)
                }
                frame #4 {
                  n99 = Negate(x=w244) -> (-x=w243:dbl)
                  n100 = call "Z Go.vi"("Increment"=TRUE, "Return Immediately"=FALSE, "Speed In"=w242, "Position In"=w243, "Gantry In"=w241) -> ("Gantry Out"=w240:refnum<k24>)  [unwired: 3 in, 3 out]
                }
              }
              n101 = Delete From Array(array=w170, length=1, index=0) -> (array with subset deleted=w169:T3)  [unwired: 1 out]
              n102 = Build Array(w175, u32 0 ("element")) -> (w172:u32[])
              n103 = disable-structure shown="Enabled" {
                disable-tunnel: w173 -> [w199 _]
                disable-tunnel: w172 -> [w198 w200]
                disable-tunnel: [w197 w200] -> w171
                frame Disabled {
                  n104 = Build Array (concatenate)(w199, w198) -> (w197:u32[])
                }
                frame Enabled {
                }
              }
            }
            frame "Circle" {
              # "Enabled This 1-23-2023"
              n105 = flat-sequence {
                tunnel: [w292] -> w279
                tunnel: w274 -> [w293]
                tunnel: w261 -> [w294]
                tunnel: w263 -> [w295]
                tunnel: w262 -> [w291]
                tunnel: [w290] -> w257
                tunnel: [w308] -> w285
                tunnel: [w307] -> w280
                tunnel: w279 -> [w307]
                tunnel: [w306] -> w258
                tunnel: w257 -> [w306]
                tunnel: w285 -> [w318]
                tunnel: [w318] -> w284
                tunnel: w280 -> [w316]
                tunnel: [w315] -> w278
                tunnel: w265 -> [w314]
                tunnel: w264 -> [w313]
                tunnel: [w317] -> w259
                tunnel: w258 -> [w317]
                tunnel: [w312] -> w254
                tunnel: [w311] -> w251
                tunnel: w284 -> [w325]
                tunnel: [w324] -> w282
                tunnel: [w323] -> w270
                tunnel: w278 -> [w322]
                tunnel: [w322] -> w277
                tunnel: [w321] -> w260
                tunnel: w259 -> [w321]
                tunnel: [w320] -> w255
                tunnel: w254 -> [w320]
                tunnel: [w319] -> w252
                tunnel: w251 -> [w319]
                tunnel: [w335] -> w283
                tunnel: w282 -> [w335]
                tunnel: w277 -> [w334]
                tunnel: [w333] -> w275
                tunnel: w273 -> [w327]
                tunnel: w272 -> [w332]
                tunnel: w271 -> [w329]
                tunnel: w260 -> [w328]
                tunnel: [w331] -> w256
                tunnel: w255 -> [w331]
                tunnel: [w330] -> w253
                tunnel: w252 -> [w330]
                tunnel: w283 -> [w340]
                tunnel: [w339] -> w269
                tunnel: [w338] -> w276
                tunnel: w275 -> [w338]
                tunnel: w256 -> [w337]
                tunnel: w253 -> [w336]
                tunnel: [w337] -> w250
                tunnel: [w336] -> w249
                tunnel: [w346] -> w281
                tunnel: w276 -> [w347]
                tunnel: w250 -> [w348]
                tunnel: w249 -> [w345]
                frame #0 {
                  n106 = case shown="False" w295 {
                    tunnel: w294 -> [w296 w303]
                    tunnel: w293 -> [w301 w305]
                    tunnel: [w300 w304] -> w292
                    tunnel: w291 -> [w299 _]
                    tunnel: [w298 w302] -> w290
                    frame False {
                      n107 = call "XY Go.vi"("return immediately"=FALSE, "Speed"=w299, "XY In"=w296, "Gantry In"=w301) -> ("XY Out"=w298:dbl[], "Gantry Out"=w300:refnum<k24>)  [unwired: 5 in, 1 out]
                    }
                    frame True {
                      n108 = call "ClearXYZTheta Go.vi"("XYZTheta In"=w303, "Gantry In"=w305) -> ("XYZTheta Out"=w302:dbl[], "Gantry Out"=w304:refnum<k24>)  [unwired: 7 in, 1 out]
                    }
                  }
                }
                frame #1 {
                  n109 = Tick Count (ms)() -> (millisecond timer value=w308:u32)
                }
                frame #2 {
                  n110 = call "Z Go.vi"("Increment"=TRUE, "Return Immediately"=FALSE, "Speed In"=w313, "Position In"=w314, "Gantry In"=w316) -> ("Speed Out"=w311:dbl, "Position Out"=w312:dbl, "Gantry Out"=w315:refnum<k24>)  [unwired: 3 in, 1 out]
                }
                frame #3 {
                  n111 = Tick Count (ms)() -> (millisecond timer value=w324:u32)
                  n112 = Subtract(x=w324, y=w325) -> (x-y=w323:u32)
                }
                frame #4 {
                  n113 = call "Circular.vi"("Direction"=w329, "return immediately"=FALSE, "Speed"=w332, "XY End"=w328, "XY Center"=w327, "Gantry In"=w334) -> ("Gantry Out"=w333:refnum<k24>)  [unwired: 4 in, 1 out]
                }
                frame #5 {
                  n114 = Tick Count (ms)() -> (millisecond timer value=w341:u32)
                  n115 = Subtract(x=w341, y=w340) -> (x-y=w339:u32)
                }
                frame #6 {
                  n116 = Negate(x=w348) -> (-x=w344:dbl)
                  n117 = call "Z Go.vi"("Increment"=TRUE, "Return Immediately"=FALSE, "Speed In"=w345, "Position In"=w344, "Gantry In"=w347) -> ("Gantry Out"=w346:refnum<k24>)  [unwired: 3 in, 3 out]
                }
              }
              n118 = Delete From Array(array=w248, length=1, index=0) -> (array with subset deleted=w247:T3)  [unwired: 1 out]
              n119 = Build Array(w270, w269) -> (w267:u32[])
              n120 = disable-structure shown="Enabled" {
                disable-tunnel: w268 -> [w288 _]
                disable-tunnel: w267 -> [w287 w289]
                disable-tunnel: [w286 w289] -> w266
                frame Enabled {
                  n121 = Build Array (concatenate)(w288, w287) -> (w286:u32[])
                }
                frame Disabled {
                }
              }
            }
            frame "Arc" {
              # "ENABLED THIS - 1/18/2023"
              n122 = flat-sequence {
                tunnel: w398 -> [w408]
                tunnel: w397 -> [w407]
                tunnel: w396 -> [w406]
                tunnel: [w405] -> w389
                tunnel: w375 -> [w404]
                tunnel: [w403] -> w359
                tunnel: w358 -> [w403]
                tunnel: w389 -> [w419]
                tunnel: [w419] -> w388
                tunnel: [w418] -> w386
                tunnel: [w417] -> w360
                tunnel: w359 -> [w417]
                tunnel: w388 -> [w429]
                tunnel: [w426] -> w391
                tunnel: w393 -> [w428]
                tunnel: w392 -> [w427]
                tunnel: [w425] -> w387
                tunnel: w386 -> [w425]
                tunnel: [w424] -> w383
                tunnel: [w423] -> w381
                tunnel: [w420] -> w361
                tunnel: w360 -> [w420]
                tunnel: w391 -> [w436]
                tunnel: [w436] -> w390
                tunnel: w387 -> [w435]
                tunnel: [w434] -> w384
                tunnel: w383 -> [w434]
                tunnel: [w433] -> w382
                tunnel: w381 -> [w433]
                tunnel: [w432] -> w380
                tunnel: [w431] -> w366
                tunnel: [w430] -> w362
                tunnel: w361 -> [w430]
                tunnel: w390 -> [w457]
                tunnel: w395 -> [w456]
                tunnel: w394 -> [w455]
                tunnel: w384 -> [w451]
                tunnel: w382 -> [w450]
                tunnel: w373 -> [w454]
                tunnel: w374 -> [w453]
                tunnel: [w452] -> w371
                tunnel: [w451] -> w369
                tunnel: [w450] -> w367
                tunnel: w366 -> [w449]
                tunnel: [w449] -> w365
                tunnel: w364 -> [w448]
                tunnel: [w447] -> w363
                tunnel: w362 -> [w446]
                tunnel: w357 -> [w445]
                tunnel: w356 -> [w443]
                tunnel: w355 -> [w444]
                tunnel: w354 -> [w442]
                tunnel: w353 -> [w441]
                tunnel: w352 -> [w440]
                tunnel: w351 -> [w439]
                tunnel: w350 -> [w438]
                tunnel: w349 -> [w437]
                tunnel: [w559] -> w379
                tunnel: [w558] -> w372
                tunnel: w371 -> [w558]
                tunnel: [w557] -> w370
                tunnel: w369 -> [w557]
                tunnel: [w556] -> w368
                tunnel: w367 -> [w556]
                tunnel: w365 -> [w554]
                tunnel: [w566] -> w385
                tunnel: w372 -> [w564]
                tunnel: w370 -> [w563]
                tunnel: w368 -> [w562]
                frame #0 {
                  n123 = case shown="True" w404 {
                    tunnel: [w413 w416] -> w405
                    tunnel: w408 -> [w412 w415]
                    tunnel: w407 -> [w409 w414]
                    tunnel: w406 -> [w411 _]
                    frame False {
                      n124 = call "XY Go.vi"("return immediately"=FALSE, "Speed"=w411, "XY In"=w409, "Gantry In"=w412) -> ("Gantry Out"=w413:refnum<k24>)  [unwired: 5 in, 2 out]
                    }
                    frame True {
                      n125 = call "ClearXYZTheta Go.vi"("XYZTheta In"=w414, "Gantry In"=w415) -> ("Gantry Out"=w416:refnum<k24>)  [unwired: 7 in, 2 out]
                    }
                  }
                }
                frame #1 {
                  n126 = Tick Count (ms)() -> (millisecond timer value=w418:u32)
                }
                frame #2 {
                  n127 = call "Z Go.vi"("Increment"=TRUE, "Return Immediately"=FALSE, "Speed In"=w427, "Position In"=w428, "Gantry In"=w429) -> ("Speed Out"=w423:dbl, "Position Out"=w424:dbl, "Gantry Out"=w426:refnum<k24>)  [unwired: 3 in, 1 out]
                }
                frame #3 {
                  n128 = Tick Count (ms)() -> (millisecond timer value=w431:u32)
                  n129 = Subtract(x=w431, y=w435) -> (x-y=w432:u32)
                }
                frame #4 {
                  n130 = case shown="True" w444 {
                    tunnel: w457 -> [w469 w553]
                    tunnel: w456 -> [w467 w552]
                    tunnel: w455 -> [w472 w551]
                    tunnel: w454 -> [w471 w550]
                    tunnel: w453 -> [w470 w549]
                    tunnel: [w468 w548] -> w452
                    tunnel: w448 -> [w474 w544]
                    tunnel: [w473 w543] -> w447
                    tunnel: w446 -> [w466 _]
                    tunnel: w445 -> [w465 _]
                    tunnel: w443 -> [w464 _]
                    tunnel: w442 -> [w463 _]
                    tunnel: w441 -> [w462 _]
                    tunnel: w440 -> [w461 _]
                    tunnel: w439 -> [w460 _]
                    tunnel: w438 -> [w459 _]
                    tunnel: w437 -> [w458 _]
                    frame True {
                      # "direction"
                      # "center"
                      # "end"
                      n131 = case shown="True" w464 {
                        tunnel: w474 -> [w476 w542]
                        tunnel: [w475 w539] -> w473
                        tunnel: w472 -> [w490 w538]
                        tunnel: w471 -> [w485 w531]
                        tunnel: w470 -> [w486 w530]
                        tunnel: w469 -> [w488 w537]
                        tunnel: [w487 w535] -> w468
                        tunnel: w467 -> [w489 w534]
                        tunnel: w466 -> [w484 _]
                        tunnel: w465 -> [w483 _]
                        tunnel: w463 -> [w482 w529]
                        tunnel: w462 -> [w481 w528]
                        tunnel: w461 -> [w480 _]
                        tunnel: w460 -> [w479 _]
                        tunnel: w459 -> [w478 _]
                        tunnel: w458 -> [w477 _]
                        frame True {
                          n132 = case shown="True" w484 {
                            tunnel: w490 -> [w502 w527]
                            tunnel: w489 -> [w503 w512]
                            tunnel: w488 -> [w507 w520]
                            tunnel: [w504 w516] -> w487
                            tunnel: w486 -> [w501 w525]
                            tunnel: w485 -> [w500 w526]
                            tunnel: w483 -> [_ _]
                            tunnel: w482 -> [w498 w523]
                            tunnel: w481 -> [w497 w524]
                            tunnel: w480 -> [w496 w522]
                            tunnel: w479 -> [w495 w521]
                            tunnel: w478 -> [_ w515]
                            tunnel: w477 -> [_ w514]
                            tunnel: w476 -> [w492 w511]
                            tunnel: [w491 w510] -> w475
                            frame False {
                              w499 = FALSE
                              n133 = call "Circular.vi"("Direction"=w502, "return immediately"=w499, "Speed"=w503, "XY End"=w501, "XY Center"=w500, "Gantry In"=w507) -> ("Gantry Out"=w506:refnum<k24>)  [unwired: 4 in, 1 out]
                              n134 = call "Circular.vi"("Direction"=w502, "return immediately"=w499, "Speed"=w503, "XY End"=w497, "XY Center"=w498, "Gantry In"=w506) -> ("Gantry Out"=w505:refnum<k24>)  [unwired: 4 in, 1 out]
                              n135 = call "Circular.vi"("Direction"=w502, "return immediately"=w499, "Speed"=w503, "XY End"=w496, "XY Center"=w495, "Gantry In"=w505) -> ("Gantry Out"=w504:refnum<k24>)  [unwired: 4 in, 1 out]
                              n136 = Delete From Array(array=w492, length=3, index=0) -> (array with subset deleted=w491:T3)  [unwired: 1 out]
                            }
                            frame True {
                              w513 = FALSE
                              n137 = Delete From Array(array=w511, length=4, index=0) -> (array with subset deleted=w510:T3)  [unwired: 1 out]
                              n138 = call "Circular.vi"("Direction"=w527, "return immediately"=w513, "Speed"=w512, "XY End"=w525, "XY Center"=w526, "Gantry In"=w520) -> ("Gantry Out"=w519:refnum<k24>)  [unwired: 4 in, 1 out]
                              n139 = call "Circular.vi"("Direction"=w527, "return immediately"=w513, "Speed"=w512, "XY End"=w524, "XY Center"=w523, "Gantry In"=w519) -> ("Gantry Out"=w518:refnum<k24>)  [unwired: 4 in, 1 out]
                              n140 = call "Circular.vi"("Direction"=w527, "return immediately"=w513, "Speed"=w512, "XY End"=w522, "XY Center"=w521, "Gantry In"=w518) -> ("Gantry Out"=w517:refnum<k24>)  [unwired: 4 in, 1 out]
                              n141 = call "Circular.vi"("Direction"=w527, "return immediately"=w513, "Speed"=w512, "XY End"=w515, "XY Center"=w514, "Gantry In"=w517) -> ("Gantry Out"=w516:refnum<k24>)  [unwired: 4 in, 1 out]
                            }
                          }
                        }
                        frame False {
                          n142 = call "Circular.vi"("Direction"=w538, "return immediately"=FALSE, "Speed"=w534, "XY End"=w530, "XY Center"=w531, "Gantry In"=w537) -> ("Gantry Out"=w536:refnum<k24>)  [unwired: 4 in, 1 out]
                          n143 = call "Circular.vi"("Direction"=w538, "return immediately"=FALSE, "Speed"=w534, "XY End"=w528, "XY Center"=w529, "Gantry In"=w536) -> ("Gantry Out"=w535:refnum<k24>)  [unwired: 4 in, 1 out]
                          n144 = Delete From Array(array=w542, length=2, index=0) -> (array with subset deleted=w539:T3)  [unwired: 1 out]
                        }
                      }
                    }
                    frame False {
                      # "end"
                      # "center"
                      # "direction"
                      n145 = call "Circular.vi"("Direction"=w551, "return immediately"=FALSE, "Speed"=w552, "XY End"=w549, "XY Center"=w550, "Gantry In"=w553) -> ("Gantry Out"=w548:refnum<k24>)  [unwired: 4 in, 1 out]
                      n146 = Delete From Array(array=w544, length=1, index=0) -> (array with subset deleted=w543:T3)  [unwired: 1 out]
                    }
                  }
                }
                frame #5 {
                  n147 = Tick Count (ms)() -> (millisecond timer value=w555:u32)
                  n148 = Subtract(x=w555, y=w554) -> (x-y=w559:u32)
                }
                frame #6 {
                  n149 = Negate(x=w563) -> (-x=w565:dbl)
                  n150 = call "Z Go.vi"("Increment"=TRUE, "Return Immediately"=FALSE, "Speed In"=w562, "Position In"=w565, "Gantry In"=w564) -> ("Gantry Out"=w566:refnum<k24>)  [unwired: 3 in, 3 out]
                }
              }
              n151 = Build Array "Build Array"(w380, w379) -> (w378:u32[])
              n152 = disable-structure shown="Enabled" {
                disable-tunnel: w378 -> [w401 w402]
                disable-tunnel: w377 -> [w400 _]
                disable-tunnel: [w399 w402] -> w376
                frame Enabled {
                  n153 = Build Array (concatenate) "Build Array"(w401, w400) -> (w399:u32[])
                }
                frame Disabled {
                }
              }
            }
            frame "Line" {
              n154 = flat-sequence {
                tunnel: w626 -> [w635]
                tunnel: w625 -> [w631]
                tunnel: w624 -> [w634]
                tunnel: w623 -> [w633]
                tunnel: [w632] -> w622
                tunnel: w622 -> [w644]
                tunnel: [w644] -> w621
                tunnel: [w645] -> w617
                tunnel: w621 -> [w654]
                tunnel: w620 -> [w653]
                tunnel: w619 -> [w652]
                tunnel: [w651] -> w618
                tunnel: w617 -> [w651]
                tunnel: [w650] -> w615
                tunnel: [w649] -> w606
                tunnel: [w648] -> w602
                tunnel: w618 -> [w660]
                tunnel: [w659] -> w599
                tunnel: [w658] -> w616
                tunnel: w615 -> [w658]
                tunnel: [w657] -> w612
                tunnel: [w656] -> w607
                tunnel: w606 -> [w656]
                tunnel: [w655] -> w603
                tunnel: w602 -> [w655]
                tunnel: w616 -> [w694]
                tunnel: w614 -> [w693]
                tunnel: [w692] -> w613
                tunnel: w612 -> [w692]
                tunnel: [w691] -> w610
                tunnel: [w690] -> w608
                tunnel: w607 -> [w690]
                tunnel: [w689] -> w604
                tunnel: w603 -> [w689]
                tunnel: w595 -> [w688]
                tunnel: w594 -> [w687]
                tunnel: w593 -> [w686]
                tunnel: w592 -> [w683]
                tunnel: w591 -> [w685]
                tunnel: [w684] -> w590
                tunnel: w589 -> [w682]
                tunnel: w588 -> [w681]
                tunnel: w587 -> [w680]
                tunnel: w586 -> [_]
                tunnel: w585 -> [w679]
                tunnel: w584 -> [w678]
                tunnel: w583 -> [w677]
                tunnel: w582 -> [w676]
                tunnel: w581 -> [w675]
                tunnel: w580 -> [w674]
                tunnel: w579 -> [w673]
                tunnel: w578 -> [w672]
                tunnel: w577 -> [w671]
                tunnel: w576 -> [w670]
                tunnel: w575 -> [w669]
                tunnel: w574 -> [w668]
                tunnel: w573 -> [w667]
                tunnel: w572 -> [w666]
                tunnel: w571 -> [w665]
                tunnel: w570 -> [w664]
                tunnel: w569 -> [w663]
                tunnel: w568 -> [w662]
                tunnel: w567 -> [w661]
                tunnel: w613 -> [w1231]
                tunnel: [w1230] -> w601
                tunnel: [w1229] -> w611
                tunnel: w610 -> [w1229]
                tunnel: [w1228] -> w609
                tunnel: w608 -> [w1228]
                tunnel: [w1227] -> w605
                tunnel: w604 -> [w1227]
                tunnel: w611 -> [w1239]
                tunnel: w609 -> [w1238]
                tunnel: w605 -> [w1236]
                tunnel: [w1235] -> w600
                frame #0 {
                  n155 = case shown="True" w633 {
                    tunnel: w635 -> [w640 w643]
                    tunnel: w634 -> [w639 _]
                    tunnel: [w638 w642] -> w632
                    tunnel: w631 -> [w637 w641]
                    frame False {
                      n156 = call "XY Go.vi"("return immediately"=FALSE, "Speed"=w639, "XY In"=w637, "Gantry In"=w640) -> ("Gantry Out"=w638:refnum<k24>)  [unwired: 5 in, 2 out]
                    }
                    frame True {
                      n157 = call "ClearXYZTheta Go.vi"("XYZTheta In"=w641, "Gantry In"=w643) -> ("Gantry Out"=w642:refnum<k24>)  [unwired: 7 in, 2 out]
                    }
                  }
                }
                frame #1 {
                  n158 = Tick Count (ms)() -> (millisecond timer value=w645:u32)
                }
                frame #2 {
                  # "ok"
                  n159 = call "Z Go.vi"("Increment"=TRUE, "Return Immediately"=FALSE, "Speed In"=w652, "Position In"=w653, "Gantry In"=w654) -> ("Speed Out"=w648:dbl, "Position Out"=w649:dbl, "Gantry Out"=w650:refnum<k24>)  [unwired: 3 in, 1 out]
                }
                frame #3 {
                  n160 = Tick Count (ms)() -> (millisecond timer value=w657:u32)
                  n161 = Subtract(x=w657, y=w660) -> (x-y=w659:u32)
                }
                frame #4 {
                  n162 = case shown="True" w687 {
                    tunnel: w694 -> [w701 w733]
                    tunnel: w693 -> [w703 w732]
                    tunnel: [w700 w731] -> w691
                    tunnel: w688 -> [w702 w730]
                    tunnel: w686 -> [_ w729]
                    tunnel: w683 -> [_ w728]
                    tunnel: w685 -> [w698 w727]
                    tunnel: [w697 w726] -> w684
                    tunnel: w682 -> [_ w725]
                    tunnel: w681 -> [_ w724]
                    tunnel: w680 -> [_ w723]
                    tunnel: w679 -> [_ w722]
                    tunnel: w678 -> [_ w721]
                    tunnel: w677 -> [_ w720]
                    tunnel: w676 -> [_ w719]
                    tunnel: w675 -> [_ w718]
                    tunnel: w674 -> [_ w717]
                    tunnel: w673 -> [_ w716]
                    tunnel: w672 -> [_ w715]
                    tunnel: w671 -> [_ w714]
                    tunnel: w670 -> [_ w713]
                    tunnel: w669 -> [_ w712]
                    tunnel: w668 -> [_ w711]
                    tunnel: w667 -> [_ w710]
                    tunnel: w666 -> [_ w709]
                    tunnel: w665 -> [_ w708]
                    tunnel: w664 -> [_ w707]
                    tunnel: w663 -> [_ w706]
                    tunnel: w662 -> [_ w705]
                    tunnel: w661 -> [_ w704]
                    frame False {
                      n163 = call "XY Go.vi"("return immediately"=FALSE, "Speed"=w703, "XY In"=w702, "Gantry In"=w701) -> ("Gantry Out"=w700:refnum<k24>)  [unwired: 5 in, 2 out]
                      n164 = Delete From Array(array=w698, length=1, index=0) -> (array with subset deleted=w697:T3)  [unwired: 1 out]
                    }
                    frame True {
                      n165 = case shown="True" w729 {
                        tunnel: w733 -> [w745 w771]
                        tunnel: w732 -> [w743 w773]
                        tunnel: [w740 w770] -> w731
                        tunnel: w730 -> [w744 w772]
                        tunnel: w728 -> [_ _]
                        tunnel: w727 -> [w739 w769]
                        tunnel: [w738 w768] -> w726
                        tunnel: w725 -> [w734 w767]
                        tunnel: w724 -> [_ w766]
                        tunnel: w723 -> [_ w765]
                        tunnel: w722 -> [_ w764]
                        tunnel: w721 -> [_ w763]
                        tunnel: w720 -> [_ w762]
                        tunnel: w719 -> [_ w761]
                        tunnel: w718 -> [_ w760]
                        tunnel: w717 -> [_ w759]
                        tunnel: w716 -> [_ w758]
                        tunnel: w715 -> [_ w757]
                        tunnel: w714 -> [_ w756]
                        tunnel: w713 -> [_ w755]
                        tunnel: w712 -> [_ w754]
                        tunnel: w711 -> [_ w753]
                        tunnel: w710 -> [_ w752]
                        tunnel: w709 -> [_ w751]
                        tunnel: w708 -> [_ w750]
                        tunnel: w707 -> [_ w749]
                        tunnel: w706 -> [_ w748]
                        tunnel: w705 -> [_ w747]
                        tunnel: w704 -> [_ w746]
                        frame False {
                          n166 = Delete From Array(array=w739, length=2, index=0) -> (array with subset deleted=w738:T3)  [unwired: 1 out]
                          n167 = call "XY Go.vi"("return immediately"=FALSE, "Speed"=w743, "XY In"=w744, "Gantry In"=w745) -> ("Gantry Out"=w741:refnum<k24>)  [unwired: 5 in, 2 out]
                          n168 = call "XY Go.vi"("return immediately"=FALSE, "Speed"=w743, "XY In"=w734, "Gantry In"=w741) -> ("Gantry Out"=w740:refnum<k24>)  [unwired: 5 in, 2 out]
                        }
                        frame True {
                          # "#8"
                          # "#7"
                          # "#6"
                          # "#5"
                          # "#4"
                          # "#3"
                          # "#1"
                          # "#2"
                          n169 = case shown="True" w765 {
                            tunnel: w773 -> [w775 w808]
                            tunnel: w772 -> [w786 w809]
                            tunnel: w771 -> [w785 w811]
                            tunnel: [w777 w810] -> w770
                            tunnel: w769 -> [w784 w813]
                            tunnel: [w783 w812] -> w768
                            tunnel: w767 -> [w776 w807]
                            tunnel: w766 -> [w774 w806]
                            tunnel: w764 -> [_ w805]
                            tunnel: w763 -> [_ w804]
                            tunnel: w762 -> [_ w803]
                            tunnel: w761 -> [_ w802]
                            tunnel: w760 -> [_ w801]
                            tunnel: w759 -> [_ w800]
                            tunnel: w758 -> [_ w799]
                            tunnel: w757 -> [_ w798]
                            tunnel: w756 -> [_ w797]
                            tunnel: w755 -> [_ w796]
                            tunnel: w754 -> [_ w795]
                            tunnel: w753 -> [_ w794]
                            tunnel: w752 -> [_ w793]
                            tunnel: w751 -> [_ w792]
                            tunnel: w750 -> [_ w791]
                            tunnel: w749 -> [_ w790]
                            tunnel: w748 -> [_ w789]
                            tunnel: w747 -> [_ w788]
                            tunnel: w746 -> [_ w787]
                            frame False {
                              n170 = call "XY Go.vi"("return immediately"=FALSE, "Speed"=w775, "XY In"=w786, "Gantry In"=w785) -> ("Gantry Out"=w779:refnum<k24>)  [unwired: 5 in, 2 out]
                              n171 = call "XY Go.vi"("Speed"=w775, "XY In"=w776, "Gantry In"=w779) -> ("Gantry Out"=w778:refnum<k24>)  [unwired: 6 in, 2 out]
                              n172 = Delete From Array(array=w784, length=3, index=0) -> (array with subset deleted=w783:T3)  [unwired: 1 out]
                              n173 = call "XY Go.vi"("Speed"=w775, "XY In"=w774, "Gantry In"=w778) -> ("Gantry Out"=w777:refnum<k24>)  [unwired: 6 in, 2 out]
                            }
                            frame True {
                              n174 = case shown="True" w788 {
                                tunnel: [w817 w854] -> w812
                                tunnel: w813 -> [w818 w853]
                                tunnel: w811 -> [w828 w852]
                                tunnel: [w824 w851] -> w810
                                tunnel: w809 -> [w823 w849]
                                tunnel: w808 -> [w822 w850]
                                tunnel: w807 -> [w821 w848]
                                tunnel: w806 -> [w820 w847]
                                tunnel: w805 -> [w819 w846]
                                tunnel: w804 -> [_ w845]
                                tunnel: w803 -> [_ w844]
                                tunnel: w802 -> [_ w843]
                                tunnel: w801 -> [_ w842]
                                tunnel: w800 -> [_ w841]
                                tunnel: w799 -> [_ w840]
                                tunnel: w798 -> [_ w839]
                                tunnel: w797 -> [_ w838]
                                tunnel: w796 -> [_ w837]
                                tunnel: w795 -> [_ w836]
                                tunnel: w794 -> [_ w835]
                                tunnel: w793 -> [_ w834]
                                tunnel: w792 -> [_ w833]
                                tunnel: w791 -> [_ w832]
                                tunnel: w790 -> [_ w831]
                                tunnel: w789 -> [_ w830]
                                tunnel: w787 -> [_ w829]
                                frame False {
                                w814 = FALSE
                                n175 = call "XY Go.vi"("return immediately"=w814, "Speed"=w822, "XY In"=w823, "Gantry In"=w828) -> ("Gantry Out"=w827:refnum<k24>)  [unwired: 5 in, 2 out]
                                n176 = Delete From Array(array=w818, length=4, index=0) -> (array with subset deleted=w817:T3)  [unwired: 1 out]
                                n177 = call "XY Go.vi"("return immediately"=w814, "Speed"=w822, "XY In"=w821, "Gantry In"=w827) -> ("Gantry Out"=w826:refnum<k24>)  [unwired: 5 in, 2 out]
                                n178 = call "XY Go.vi"("return immediately"=w814, "Speed"=w822, "XY In"=w820, "Gantry In"=w826) -> ("Gantry Out"=w825:refnum<k24>)  [unwired: 5 in, 2 out]
                                n179 = call "XY Go.vi"("return immediately"=w814, "Speed"=w822, "XY In"=w819, "Gantry In"=w825) -> ("Gantry Out"=w824:refnum<k24>)  [unwired: 5 in, 2 out]
                                }
                                frame True {
                                n180 = case shown="True" w829 {
                                tunnel: [w870 w893] -> w854
                                tunnel: w853 -> [w871 w894]
                                tunnel: w852 -> [w867 w896]
                                tunnel: [w862 w895] -> w851
                                tunnel: w850 -> [w857 w892]
                                tunnel: w849 -> [w861 w891]
                                tunnel: w848 -> [w860 w890]
                                tunnel: w847 -> [w859 w888]
                                tunnel: w846 -> [w858 w889]
                                tunnel: w845 -> [w856 w887]
                                tunnel: w844 -> [_ w886]
                                tunnel: w843 -> [_ w885]
                                tunnel: w842 -> [_ w884]
                                tunnel: w841 -> [_ w883]
                                tunnel: w840 -> [_ w882]
                                tunnel: w839 -> [_ w881]
                                tunnel: w838 -> [_ w880]
                                tunnel: w837 -> [_ w879]
                                tunnel: w836 -> [_ w878]
                                tunnel: w835 -> [_ w877]
                                tunnel: w834 -> [_ w876]
                                tunnel: w833 -> [_ w875]
                                tunnel: w832 -> [_ w874]
                                tunnel: w831 -> [_ w873]
                                tunnel: w830 -> [_ w872]
                                frame False {
                                w855 = FALSE
                                n181 = call "XY Go.vi"("return immediately"=w855, "Speed"=w857, "XY In"=w861, "Gantry In"=w867) -> ("Gantry Out"=w866:refnum<k24>)  [unwired: 5 in, 2 out]
                                n182 = Delete From Array(array=w871, length=5, index=0) -> (array with subset deleted=w870:T3)  [unwired: 1 out]
                                n183 = call "XY Go.vi"("return immediately"=w855, "Speed"=w857, "XY In"=w860, "Gantry In"=w866) -> ("Gantry Out"=w865:refnum<k24>)  [unwired: 5 in, 2 out]
                                n184 = call "XY Go.vi"("return immediately"=w855, "Speed"=w857, "XY In"=w859, "Gantry In"=w865) -> ("Gantry Out"=w864:refnum<k24>)  [unwired: 5 in, 2 out]
                                n185 = call "XY Go.vi"("return immediately"=w855, "Speed"=w857, "XY In"=w858, "Gantry In"=w864) -> ("Gantry Out"=w863:refnum<k24>)  [unwired: 5 in, 2 out]
                                n186 = call "XY Go.vi"("return immediately"=w855, "Speed"=w857, "XY In"=w856, "Gantry In"=w863) -> ("Gantry Out"=w862:refnum<k24>)  [unwired: 5 in, 2 out]
                                }
                                frame True {
                                n187 = case shown="True" w872 {
                                tunnel: w896 -> [w915 w937]
                                tunnel: [w909 w936] -> w895
                                tunnel: w894 -> [w906 w939]
                                tunnel: [w905 w935] -> w893
                                tunnel: w892 -> [w904 w934]
                                tunnel: w891 -> [w903 w938]
                                tunnel: w890 -> [w902 w933]
                                tunnel: w889 -> [w901 w916]
                                tunnel: w888 -> [w900 w917]
                                tunnel: w887 -> [w899 w932]
                                tunnel: w886 -> [w898 w931]
                                tunnel: w885 -> [_ w930]
                                tunnel: w884 -> [_ w929]
                                tunnel: w883 -> [_ w928]
                                tunnel: w882 -> [_ w927]
                                tunnel: w881 -> [_ w926]
                                tunnel: w880 -> [_ w925]
                                tunnel: w879 -> [_ w924]
                                tunnel: w878 -> [_ w923]
                                tunnel: w877 -> [_ w922]
                                tunnel: w876 -> [_ w921]
                                tunnel: w875 -> [_ w920]
                                tunnel: w874 -> [_ w919]
                                tunnel: w873 -> [_ w918]
                                frame False {
                                w897 = FALSE
                                n188 = call "XY Go.vi"("return immediately"=w897, "Speed"=w904, "XY In"=w903, "Gantry In"=w915) -> ("Gantry Out"=w914:refnum<k24>)  [unwired: 5 in, 2 out]
                                n189 = call "XY Go.vi"("return immediately"=w897, "Speed"=w904, "XY In"=w902, "Gantry In"=w914) -> ("Gantry Out"=w913:refnum<k24>)  [unwired: 5 in, 2 out]
                                n190 = call "XY Go.vi"("return immediately"=w897, "Speed"=w904, "XY In"=w901, "Gantry In"=w913) -> ("Gantry Out"=w912:refnum<k24>)  [unwired: 5 in, 2 out]
                                n191 = Delete From Array(array=w906, length=6, index=0) -> (array with subset deleted=w905:T3)  [unwired: 1 out]
                                n192 = call "XY Go.vi"("return immediately"=w897, "Speed"=w904, "XY In"=w900, "Gantry In"=w912) -> ("Gantry Out"=w911:refnum<k24>)  [unwired: 5 in, 2 out]
                                n193 = call "XY Go.vi"("return immediately"=w897, "Speed"=w904, "XY In"=w899, "Gantry In"=w911) -> ("Gantry Out"=w910:refnum<k24>)  [unwired: 5 in, 2 out]
                                n194 = call "XY Go.vi"("return immediately"=w897, "Speed"=w904, "XY In"=w898, "Gantry In"=w910) -> ("Gantry Out"=w909:refnum<k24>)  [unwired: 5 in, 2 out]
                                }
                                frame True {
                                # "#5"
                                # "#4"
                                n195 = case shown="True" w923 {
                                tunnel: w939 -> [w959 w982]
                                tunnel: w938 -> [w956 w977]
                                tunnel: w937 -> [w955 w980]
                                tunnel: [w948 w979] -> w936
                                tunnel: [w947 w981] -> w935
                                tunnel: w934 -> [w946 w978]
                                tunnel: w933 -> [w945 w976]
                                tunnel: w916 -> [w941 w975]
                                tunnel: w917 -> [w940 w974]
                                tunnel: w932 -> [w944 w973]
                                tunnel: w931 -> [w943 w972]
                                tunnel: w930 -> [w942 w971]
                                tunnel: w929 -> [_ w970]
                                tunnel: w928 -> [_ w969]
                                tunnel: w927 -> [_ w968]
                                tunnel: w926 -> [_ w967]
                                tunnel: w925 -> [_ w966]
                                tunnel: w924 -> [_ w965]
                                tunnel: w922 -> [_ w964]
                                tunnel: w921 -> [_ w963]
                                tunnel: w920 -> [_ w962]
                                tunnel: w919 -> [_ w961]
                                tunnel: w918 -> [_ w960]
                                frame False {
                                n196 = call "XY Go.vi"("Speed"=w946, "XY In"=w956, "Gantry In"=w955) -> ("Gantry Out"=w954:refnum<k24>)  [unwired: 6 in, 2 out]
                                n197 = call "XY Go.vi"("Speed"=w946, "XY In"=w945, "Gantry In"=w954) -> ("Gantry Out"=w953:refnum<k24>)  [unwired: 6 in, 2 out]
                                n198 = call "XY Go.vi"("Speed"=w946, "XY In"=w940, "Gantry In"=w953) -> ("Gantry Out"=w952:refnum<k24>)  [unwired: 6 in, 2 out]
                                n199 = Delete From Array(array=w959, length=7, index=0) -> (array with subset deleted=w947:T3)  [unwired: 1 out]
                                n200 = call "XY Go.vi"("Speed"=w946, "XY In"=w941, "Gantry In"=w952) -> ("Gantry Out"=w951:refnum<k24>)  [unwired: 6 in, 2 out]
                                n201 = call "XY Go.vi"("Speed"=w946, "XY In"=w944, "Gantry In"=w951) -> ("Gantry Out"=w950:refnum<k24>)  [unwired: 6 in, 2 out]
                                n202 = call "XY Go.vi"("Speed"=w946, "XY In"=w943, "Gantry In"=w950) -> ("Gantry Out"=w949:refnum<k24>)  [unwired: 6 in, 2 out]
                                n203 = call "XY Go.vi"("Speed"=w946, "XY In"=w942, "Gantry In"=w949) -> ("Gantry Out"=w948:refnum<k24>)  [unwired: 6 in, 2 out]
                                }
                                frame True {
                                n204 = case shown="True" w964 {
                                tunnel: w982 -> [w1004 w1026]
                                tunnel: [w1003 w1023] -> w981
                                tunnel: w980 -> [w1000 w1025]
                                tunnel: [w992 w1024] -> w979
                                tunnel: w978 -> [w991 w1022]
                                tunnel: w977 -> [w990 w1021]
                                tunnel: w976 -> [w989 w1020]
                                tunnel: w975 -> [w983 w1019]
                                tunnel: w974 -> [w984 w1018]
                                tunnel: w973 -> [w988 w1017]
                                tunnel: w972 -> [w987 w1016]
                                tunnel: w971 -> [w986 w1015]
                                tunnel: w970 -> [w985 w1014]
                                tunnel: w969 -> [_ w1013]
                                tunnel: w968 -> [_ w1012]
                                tunnel: w967 -> [_ w1011]
                                tunnel: w966 -> [_ w1010]
                                tunnel: w965 -> [_ w1009]
                                tunnel: w963 -> [_ w1008]
                                tunnel: w962 -> [_ w1007]
                                tunnel: w961 -> [_ w1006]
                                tunnel: w960 -> [_ w1005]
                                frame False {
                                n205 = call "XY Go.vi"("Speed"=w991, "XY In"=w990, "Gantry In"=w1000) -> ("Gantry Out"=w999:refnum<k24>)  [unwired: 6 in, 2 out]
                                n206 = call "XY Go.vi"("Speed"=w991, "XY In"=w989, "Gantry In"=w999) -> ("Gantry Out"=w998:refnum<k24>)  [unwired: 6 in, 2 out]
                                n207 = call "XY Go.vi"("Speed"=w991, "XY In"=w984, "Gantry In"=w998) -> ("Gantry Out"=w997:refnum<k24>)  [unwired: 6 in, 2 out]
                                n208 = Delete From Array(array=w1004, length=8, index=0) -> (array with subset deleted=w1003:T3)  [unwired: 1 out]
                                n209 = call "XY Go.vi"("Speed"=w991, "XY In"=w983, "Gantry In"=w997) -> ("Gantry Out"=w996:refnum<k24>)  [unwired: 6 in, 2 out]
                                n210 = call "XY Go.vi"("Speed"=w991, "XY In"=w988, "Gantry In"=w996) -> ("Gantry Out"=w995:refnum<k24>)  [unwired: 6 in, 2 out]
                                n211 = call "XY Go.vi"("Speed"=w991, "XY In"=w987, "Gantry In"=w995) -> ("Gantry Out"=w994:refnum<k24>)  [unwired: 6 in, 2 out]
                                n212 = call "XY Go.vi"("Speed"=w991, "XY In"=w986, "Gantry In"=w994) -> ("Gantry Out"=w993:refnum<k24>)  [unwired: 6 in, 2 out]
                                n213 = call "XY Go.vi"("Speed"=w991, "XY In"=w985, "Gantry In"=w993) -> ("Gantry Out"=w992:refnum<k24>)  [unwired: 6 in, 2 out]
                                }
                                frame True {
                                # "#11"
                                # "#10"
                                # "#9"
                                n214 = case shown="True" w1008 {
                                tunnel: w1026 -> [w1050 w1071]
                                tunnel: w1025 -> [w1047 w1069]
                                tunnel: [w1038 w1068] -> w1024
                                tunnel: [w1037 w1070] -> w1023
                                tunnel: w1022 -> [w1036 w1067]
                                tunnel: w1021 -> [w1035 w1066]
                                tunnel: w1020 -> [w1034 w1065]
                                tunnel: w1019 -> [w1027 w1064]
                                tunnel: w1018 -> [w1028 w1063]
                                tunnel: w1017 -> [w1033 w1062]
                                tunnel: w1016 -> [w1032 w1061]
                                tunnel: w1015 -> [w1031 w1060]
                                tunnel: w1014 -> [w1030 w1059]
                                tunnel: w1013 -> [w1029 w1058]
                                tunnel: w1012 -> [_ w1057]
                                tunnel: w1011 -> [_ w1056]
                                tunnel: w1010 -> [_ w1055]
                                tunnel: w1009 -> [_ w1054]
                                tunnel: w1007 -> [_ w1053]
                                tunnel: w1006 -> [_ w1052]
                                tunnel: w1005 -> [_ w1051]
                                frame False {
                                n215 = call "XY Go.vi"("Speed"=w1036, "XY In"=w1035, "Gantry In"=w1047) -> ("Gantry Out"=w1046:refnum<k24>)  [unwired: 6 in, 2 out]
                                n216 = call "XY Go.vi"("Speed"=w1036, "XY In"=w1034, "Gantry In"=w1046) -> ("Gantry Out"=w1045:refnum<k24>)  [unwired: 6 in, 2 out]
                                n217 = call "XY Go.vi"("Speed"=w1036, "XY In"=w1028, "Gantry In"=w1045) -> ("Gantry Out"=w1044:refnum<k24>)  [unwired: 6 in, 2 out]
                                n218 = call "XY Go.vi"("Speed"=w1036, "XY In"=w1027, "Gantry In"=w1044) -> ("Gantry Out"=w1043:refnum<k24>)  [unwired: 6 in, 2 out]
                                n219 = Delete From Array(array=w1050, length=9, index=0) -> (array with subset deleted=w1037:T3)  [unwired: 1 out]
                                n220 = call "XY Go.vi"("Speed"=w1036, "XY In"=w1033, "Gantry In"=w1043) -> ("Gantry Out"=w1042:refnum<k24>)  [unwired: 6 in, 2 out]
                                n221 = call "XY Go.vi"("Speed"=w1036, "XY In"=w1032, "Gantry In"=w1042) -> ("Gantry Out"=w1041:refnum<k24>)  [unwired: 6 in, 2 out]
                                n222 = call "XY Go.vi"("Speed"=w1036, "XY In"=w1031, "Gantry In"=w1041) -> ("Gantry Out"=w1040:refnum<k24>)  [unwired: 6 in, 2 out]
                                n223 = call "XY Go.vi"("Speed"=w1036, "XY In"=w1030, "Gantry In"=w1040) -> ("Gantry Out"=w1039:refnum<k24>)  [unwired: 6 in, 2 out]
                                n224 = call "XY Go.vi"("Speed"=w1036, "XY In"=w1029, "Gantry In"=w1039) -> ("Gantry Out"=w1038:refnum<k24>)  [unwired: 6 in, 2 out]
                                }
                                frame True {
                                n225 = case shown="True" w1053 {
                                tunnel: w1071 -> [w1097 w1117]
                                tunnel: [w1096 w1116] -> w1070
                                tunnel: w1069 -> [w1093 w1112]
                                tunnel: [w1083 w1111] -> w1068
                                tunnel: w1067 -> [w1082 w1114]
                                tunnel: w1066 -> [w1081 w1115]
                                tunnel: w1065 -> [w1080 w1113]
                                tunnel: w1064 -> [w1073 w1110]
                                tunnel: w1063 -> [w1072 w1109]
                                tunnel: w1062 -> [w1079 w1108]
                                tunnel: w1061 -> [w1078 w1107]
                                tunnel: w1060 -> [w1077 w1106]
                                tunnel: w1059 -> [w1076 w1105]
                                tunnel: w1058 -> [w1075 w1104]
                                tunnel: w1057 -> [w1074 w1103]
                                tunnel: w1056 -> [_ w1102]
                                tunnel: w1055 -> [_ w1101]
                                tunnel: w1054 -> [_ w1100]
                                tunnel: w1052 -> [_ w1099]
                                tunnel: w1051 -> [_ w1098]
                                frame False {
                                n226 = call "XY Go.vi"("Speed"=w1082, "XY In"=w1081, "Gantry In"=w1093) -> ("Gantry Out"=w1092:refnum<k24>)  [unwired: 6 in, 2 out]
                                n227 = call "XY Go.vi"("Speed"=w1082, "XY In"=w1080, "Gantry In"=w1092) -> ("Gantry Out"=w1091:refnum<k24>)  [unwired: 6 in, 2 out]
                                n228 = call "XY Go.vi"("Speed"=w1082, "XY In"=w1072, "Gantry In"=w1091) -> ("Gantry Out"=w1090:refnum<k24>)  [unwired: 6 in, 2 out]
                                n229 = call "XY Go.vi"("Speed"=w1082, "XY In"=w1073, "Gantry In"=w1090) -> ("Gantry Out"=w1089:refnum<k24>)  [unwired: 6 in, 2 out]
                                n230 = Delete From Array(array=w1097, length=10, index=0) -> (array with subset deleted=w1096:T3)  [unwired: 1 out]
                                n231 = call "XY Go.vi"("Speed"=w1082, "XY In"=w1079, "Gantry In"=w1089) -> ("Gantry Out"=w1088:refnum<k24>)  [unwired: 6 in, 2 out]
                                n232 = call "XY Go.vi"("Speed"=w1082, "XY In"=w1078, "Gantry In"=w1088) -> ("Gantry Out"=w1087:refnum<k24>)  [unwired: 6 in, 2 out]
                                n233 = call "XY Go.vi"("Speed"=w1082, "XY In"=w1077, "Gantry In"=w1087) -> ("Gantry Out"=w1086:refnum<k24>)  [unwired: 6 in, 2 out]
                                n234 = call "XY Go.vi"("Speed"=w1082, "XY In"=w1076, "Gantry In"=w1086) -> ("Gantry Out"=w1085:refnum<k24>)  [unwired: 6 in, 2 out]
                                n235 = call "XY Go.vi"("Speed"=w1082, "XY In"=w1075, "Gantry In"=w1085) -> ("Gantry Out"=w1084:refnum<k24>)  [unwired: 6 in, 2 out]
                                n236 = call "XY Go.vi"("Speed"=w1082, "XY In"=w1074, "Gantry In"=w1084) -> ("Gantry Out"=w1083:refnum<k24>)  [unwired: 6 in, 2 out]
                                }
                                frame True {
                                n237 = case shown="True" w1099 {
                                tunnel: w1117 -> [w1143 w1164]
                                tunnel: [w1142 w1163] -> w1116
                                tunnel: w1115 -> [w1141 w1162]
                                tunnel: w1114 -> [w1127 w1159]
                                tunnel: w1113 -> [w1140 w1158]
                                tunnel: w1112 -> [w1139 w1161]
                                tunnel: [w1128 w1160] -> w1111
                                tunnel: w1110 -> [w1119 w1146]
                                tunnel: w1109 -> [w1118 w1147]
                                tunnel: w1108 -> [w1126 w1157]
                                tunnel: w1107 -> [w1125 w1156]
                                tunnel: w1106 -> [w1124 w1155]
                                tunnel: w1105 -> [w1123 w1154]
                                tunnel: w1104 -> [w1122 w1153]
                                tunnel: w1103 -> [w1121 w1152]
                                tunnel: w1102 -> [w1120 w1151]
                                tunnel: w1101 -> [_ w1150]
                                tunnel: w1100 -> [_ w1149]
                                tunnel: w1098 -> [_ w1148]
                                frame False {
                                n238 = call "XY Go.vi"("Speed"=w1127, "XY In"=w1141, "Gantry In"=w1139) -> ("Gantry Out"=w1138:refnum<k24>)  [unwired: 6 in, 2 out]
                                n239 = call "XY Go.vi"("Speed"=w1127, "XY In"=w1140, "Gantry In"=w1138) -> ("Gantry Out"=w1137:refnum<k24>)  [unwired: 6 in, 2 out]
                                n240 = call "XY Go.vi"("Speed"=w1127, "XY In"=w1118, "Gantry In"=w1137) -> ("Gantry Out"=w1136:refnum<k24>)  [unwired: 6 in, 2 out]
                                n241 = call "XY Go.vi"("Speed"=w1127, "XY In"=w1119, "Gantry In"=w1136) -> ("Gantry Out"=w1135:refnum<k24>)  [unwired: 6 in, 2 out]
                                n242 = call "XY Go.vi"("Speed"=w1127, "XY In"=w1126, "Gantry In"=w1135) -> ("Gantry Out"=w1134:refnum<k24>)  [unwired: 6 in, 2 out]
                                n243 = Delete From Array(array=w1143, length=11, index=0) -> (array with subset deleted=w1142:T3)  [unwired: 1 out]
                                n244 = call "XY Go.vi"("Speed"=w1127, "XY In"=w1125, "Gantry In"=w1134) -> ("Gantry Out"=w1133:refnum<k24>)  [unwired: 6 in, 2 out]
                                n245 = call "XY Go.vi"("Speed"=w1127, "XY In"=w1124, "Gantry In"=w1133) -> ("Gantry Out"=w1132:refnum<k24>)  [unwired: 6 in, 2 out]
                                n246 = call "XY Go.vi"("Speed"=w1127, "XY In"=w1123, "Gantry In"=w1132) -> ("Gantry Out"=w1131:refnum<k24>)  [unwired: 6 in, 2 out]
                                n247 = call "XY Go.vi"("Speed"=w1127, "XY In"=w1122, "Gantry In"=w1131) -> ("Gantry Out"=w1130:refnum<k24>)  [unwired: 6 in, 2 out]
                                n248 = call "XY Go.vi"("Speed"=w1127, "XY In"=w1121, "Gantry In"=w1130) -> ("Gantry Out"=w1129:refnum<k24>)  [unwired: 6 in, 2 out]
                                n249 = call "XY Go.vi"("Speed"=w1127, "XY In"=w1120, "Gantry In"=w1129) -> ("Gantry Out"=w1128:refnum<k24>)  [unwired: 6 in, 2 out]
                                }
                                frame True {
                                n250 = case shown="True" w1148 {
                                tunnel: w1164 -> [w1194 w1224]
                                tunnel: [w1193 w1223] -> w1163
                                tunnel: w1162 -> [w1190 w1222]
                                tunnel: w1161 -> [w1189 w1221]
                                tunnel: [w1177 w1208] -> w1160
                                tunnel: w1159 -> [w1176 w1198]
                                tunnel: w1158 -> [w1175 w1207]
                                tunnel: w1157 -> [w1174 w1206]
                                tunnel: w1156 -> [w1173 w1205]
                                tunnel: w1155 -> [w1172 w1204]
                                tunnel: w1154 -> [w1171 w1203]
                                tunnel: w1153 -> [w1170 w1202]
                                tunnel: w1152 -> [w1169 w1201]
                                tunnel: w1151 -> [w1168 w1200]
                                tunnel: w1150 -> [w1167 w1199]
                                tunnel: w1149 -> [_ w1197]
                                tunnel: w1146 -> [w1166 w1196]
                                tunnel: w1147 -> [w1165 w1195]
                                frame False {
                                n251 = call "XY Go.vi"("Speed"=w1176, "XY In"=w1190, "Gantry In"=w1189) -> ("Gantry Out"=w1188:refnum<k24>)  [unwired: 6 in, 2 out]
                                n252 = call "XY Go.vi"("Speed"=w1176, "XY In"=w1175, "Gantry In"=w1188) -> ("Gantry Out"=w1187:refnum<k24>)  [unwired: 6 in, 2 out]
                                n253 = call "XY Go.vi"("Speed"=w1176, "XY In"=w1165, "Gantry In"=w1187) -> ("Gantry Out"=w1186:refnum<k24>)  [unwired: 6 in, 2 out]
                                n254 = call "XY Go.vi"("Speed"=w1176, "XY In"=w1166, "Gantry In"=w1186) -> ("Gantry Out"=w1185:refnum<k24>)  [unwired: 6 in, 2 out]
                                n255 = Delete From Array(array=w1194, length=12, index=0) -> (array with subset deleted=w1193:T3)  [unwired: 1 out]
                                n256 = call "XY Go.vi"("Speed"=w1176, "XY In"=w1174, "Gantry In"=w1185) -> ("Gantry Out"=w1184:refnum<k24>)  [unwired: 6 in, 2 out]
                                n257 = call "XY Go.vi"("Speed"=w1176, "XY In"=w1173, "Gantry In"=w1184) -> ("Gantry Out"=w1183:refnum<k24>)  [unwired: 6 in, 2 out]
                                n258 = call "XY Go.vi"("Speed"=w1176, "XY In"=w1172, "Gantry In"=w1183) -> ("Gantry Out"=w1182:refnum<k24>)  [unwired: 6 in, 2 out]
                                n259 = call "XY Go.vi"("Speed"=w1176, "XY In"=w1171, "Gantry In"=w1182) -> ("Gantry Out"=w1181:refnum<k24>)  [unwired: 6 in, 2 out]
                                n260 = call "XY Go.vi"("Speed"=w1176, "XY In"=w1170, "Gantry In"=w1181) -> ("Gantry Out"=w1180:refnum<k24>)  [unwired: 6 in, 2 out]
                                n261 = call "XY Go.vi"("Speed"=w1176, "XY In"=w1169, "Gantry In"=w1180) -> ("Gantry Out"=w1179:refnum<k24>)  [unwired: 6 in, 2 out]
                                n262 = call "XY Go.vi"("Speed"=w1176, "XY In"=w1168, "Gantry In"=w1179) -> ("Gantry Out"=w1178:refnum<k24>)  [unwired: 6 in, 2 out]
                                n263 = call "XY Go.vi"("Speed"=w1176, "XY In"=w1167, "Gantry In"=w1178) -> ("Gantry Out"=w1177:refnum<k24>)  [unwired: 6 in, 2 out]
                                }
                                frame True {
                                n264 = call "XY Go.vi"("Speed"=w1198, "XY In"=w1222, "Gantry In"=w1221) -> ("Gantry Out"=w1220:refnum<k24>)  [unwired: 6 in, 2 out]
                                n265 = call "XY Go.vi"("Speed"=w1198, "XY In"=w1207, "Gantry In"=w1220) -> ("Gantry Out"=w1219:refnum<k24>)  [unwired: 6 in, 2 out]
                                n266 = call "XY Go.vi"("Speed"=w1198, "XY In"=w1195, "Gantry In"=w1219) -> ("Gantry Out"=w1218:refnum<k24>)  [unwired: 6 in, 2 out]
                                n267 = call "XY Go.vi"("Speed"=w1198, "XY In"=w1196, "Gantry In"=w1218) -> ("Gantry Out"=w1217:refnum<k24>)  [unwired: 6 in, 2 out]
                                n268 = call "XY Go.vi"("Speed"=w1198, "XY In"=w1206, "Gantry In"=w1217) -> ("Gantry Out"=w1216:refnum<k24>)  [unwired: 6 in, 2 out]
                                n269 = call "XY Go.vi"("Speed"=w1198, "XY In"=w1205, "Gantry In"=w1216) -> ("Gantry Out"=w1215:refnum<k24>)  [unwired: 6 in, 2 out]
                                n270 = Delete From Array(array=w1224, length=13, index=0) -> (array with subset deleted=w1223:T3)  [unwired: 1 out]
                                n271 = call "XY Go.vi"("Speed"=w1198, "XY In"=w1204, "Gantry In"=w1215) -> ("Gantry Out"=w1214:refnum<k24>)  [unwired: 6 in, 2 out]
                                n272 = call "XY Go.vi"("Speed"=w1198, "XY In"=w1203, "Gantry In"=w1214) -> ("Gantry Out"=w1213:refnum<k24>)  [unwired: 6 in, 2 out]
                                n273 = call "XY Go.vi"("Speed"=w1198, "XY In"=w1202, "Gantry In"=w1213) -> ("Gantry Out"=w1212:refnum<k24>)  [unwired: 6 in, 2 out]
                                n274 = call "XY Go.vi"("Speed"=w1198, "XY In"=w1201, "Gantry In"=w1212) -> ("Gantry Out"=w1211:refnum<k24>)  [unwired: 6 in, 2 out]
                                n275 = call "XY Go.vi"("Speed"=w1198, "XY In"=w1200, "Gantry In"=w1211) -> ("Gantry Out"=w1210:refnum<k24>)  [unwired: 6 in, 2 out]
                                n276 = call "XY Go.vi"("Speed"=w1198, "XY In"=w1199, "Gantry In"=w1210) -> ("Gantry Out"=w1209:refnum<k24>)  [unwired: 6 in, 2 out]
                                n277 = call "XY Go.vi"("Speed"=w1198, "XY In"=w1197, "Gantry In"=w1209) -> ("Gantry Out"=w1208:refnum<k24>)  [unwired: 6 in, 2 out]
                                }
                                }
                                }
                                }
                                }
                                }
                                }
                                }
                                }
                                }
                                }
                                }
                                }
                                }
                                }
                                }
                                }
                              }
                            }
                          }
                        }
                      }
                    }
                  }
                }
                frame #5 {
                  # "measures time\nit takes to move\nfrom P(i) to P(i+1)"
                  n278 = Tick Count (ms)() -> (millisecond timer value=w1232:u32)
                  n279 = Subtract(x=w1232, y=w1231) -> (x-y=w1230:u32)
                }
                frame #6 {
                  n280 = Negate(x=w1238) -> (-x=w1237:dbl)
                  n281 = call "Z Go.vi"("Increment"=TRUE, "Return Immediately"=FALSE, "Speed In"=w1236, "Position In"=w1237, "Gantry In"=w1239) -> ("Gantry Out"=w1235:refnum<k24>)  [unwired: 3 in, 3 out]
                }
              }
              n282 = Build Array(w599, w601) -> (w597:u32[])
              n283 = disable-structure shown="Enabled" {
                disable-tunnel: w598 -> [w629 _]
                disable-tunnel: w597 -> [w628 w630]
                disable-tunnel: [w627 w630] -> w596
                frame Disabled {
                  n284 = Build Array (concatenate)(w629, w628) -> (w627:u32[])
                }
                frame Enabled {
                }
              }
            }
          }
          n285 = Array Size(array=w115) -> (size(s)=w114:i32)
          n286 = Equal To 0?(x=w114) -> (x = 0?=w112:bool)
        }
        "Timing Data" <- w18
        n287 = in-place-cluster #1("Gantry"=w19) -> (w9:T2)
      }
    }
    frame Error {
      (unwired) T3 [] ("Dispense Steps")
    }
  }
  "error out" <- w2
  "Sensor Dispense out" <- w5
  "Control Out" <- w3
